vi "NewVSSNavigation.vi"(0 "GoTo Navigation":bool, 1 "a1":dbl=10.0, 2 "VelNearBall":dbl=1.0 format="%#_13g", 3 "output xy":dbl, 4 "IA State Output in":T2, 6 "a3":dbl=15.0, 7 "Penalty Shoot Out?":bool, 8 "PID gains Vel":T1={"proportional gain (Kc)"=0.6, "integral time (Ti, min)"=0.0, "derivative time (Td, min)"=0.0}, 9 "Test Mode":bool, 10 "Debug":bool, 11 "output inc":dbl, 13 "output angle":dbl) -> (14 "IA State Output out":T2)   [LabVIEW 2022 SP3]
uses:
  Vision_class/Old vision/SSL Detection Frame Simple Estimator Cameras VelCmd Folder/Core/AI Input.ctl
  Vision_class/Old vision/Controls/AI Robot.ctl
  Vision_class/Old vision/Controls/Functions Enum.ctl
  Vision_class/Old vision/Controls/AttackerStates.ctl
  Vision_class/Old vision/Controls/PathDests.ctl
  Vision_class/Old vision/Controls/PathDest.ctl
  VSSAttackerStates.ctl
  Vision_class/Old vision/SSL Detection Frame Simple Estimator Cameras VelCmd Folder/Core/AI Ball.ctl
  Vision_class/Old vision/SSL Detection Frame Simple Estimator Cameras VelCmd Folder/Core/Field Size.ctl
  Vision_class/Old vision/SSL Detection Frame Simple Estimator Cameras VelCmd Folder/Core/AI Judge.ctl
  Communication_class/Paths/MessageAI_State Folder/Intel/Command Enum.ctl
  Vision_class/Old vision/SSL Detection Frame Simple Estimator Cameras VelCmd Folder/Util/Events/Events.ctl
  Utilities_class/Utilities.lvclass
  Parameters_class/Project.ctl
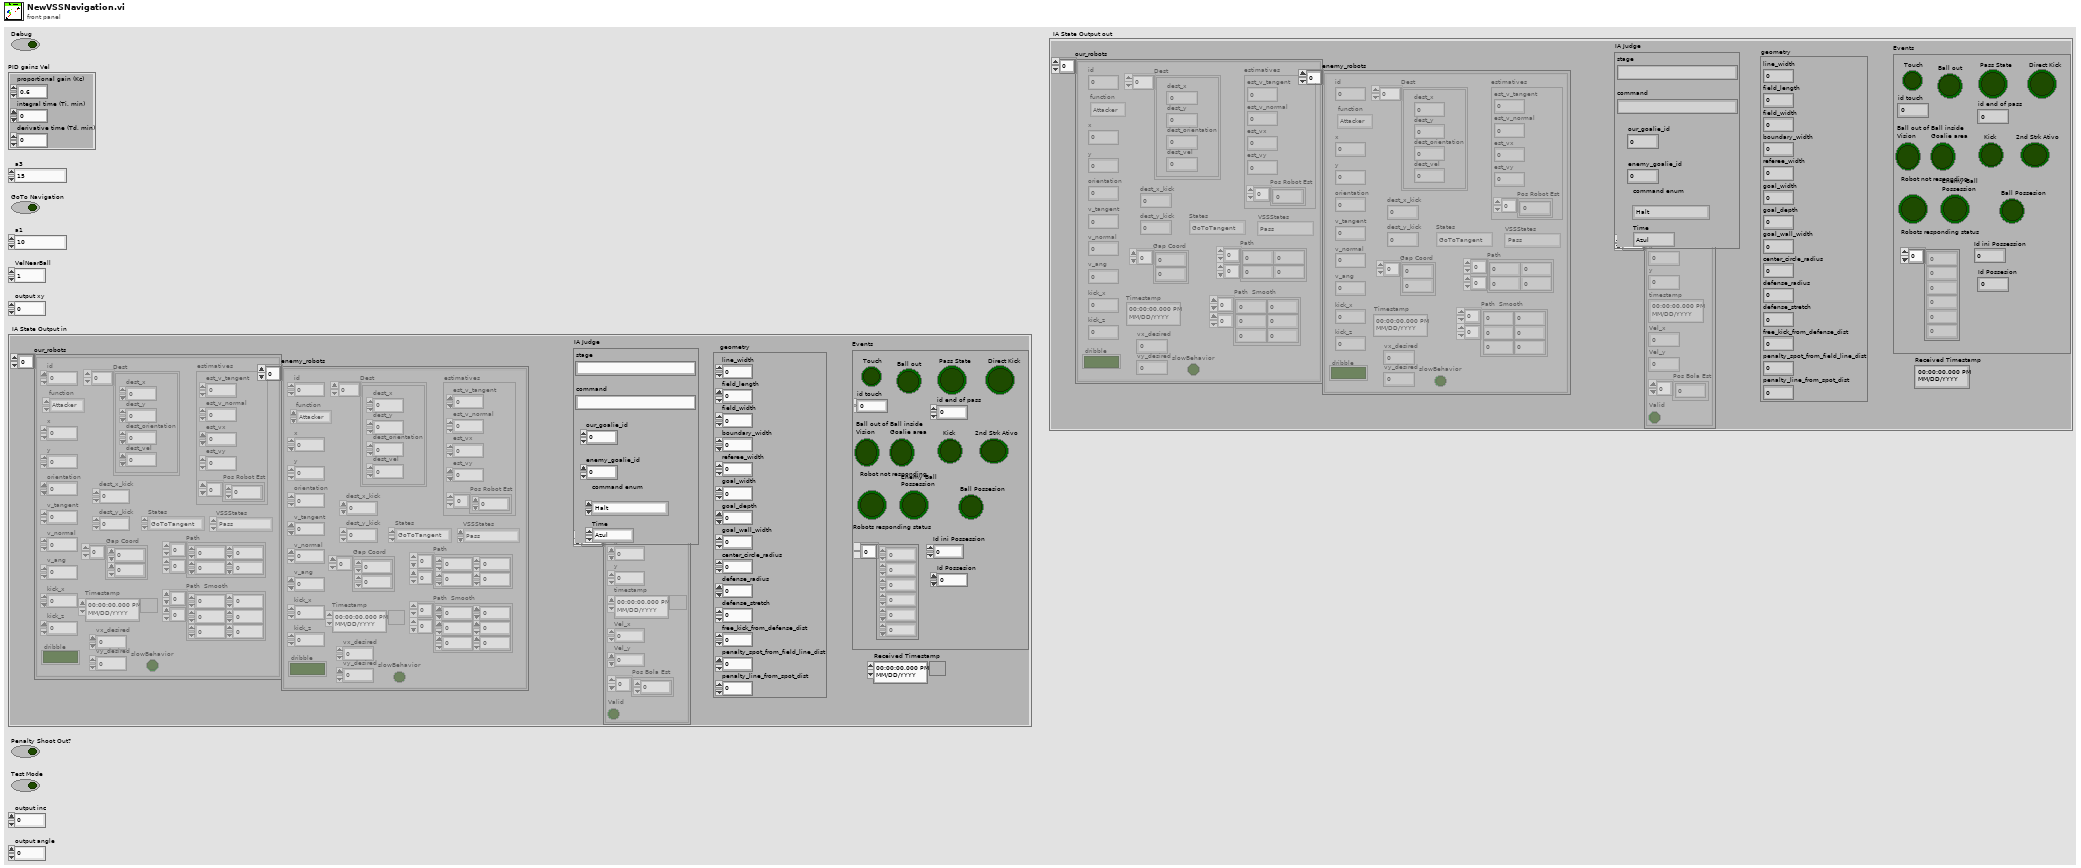
[diagram p1: front panel]
types:
  T1 = cluster{"proportional gain (Kc)":dbl, "integral time (Ti, min)":dbl, "derivative time (Td, min)":dbl}
  T2 = typedef "AI Input.ctl" = cluster{"our_robots":T3[], "enemy_robots":T3[], "balls":T9[], "geometry":T10, "IA Judge":T11, "Received Timestamp":timestamp, "Events":T13}
  T3 = typedef "AI Robot.ctl" = cluster{"id":u32, "function":T4, "x":dbl, "y":dbl, "orientation":dbl, "v_tangent":dbl, "v_normal":dbl, "v_ang":dbl, "kick_x":dbl, "kick_z":dbl, "dribble":bool, "Timestamp":timestamp, "estimatives":cluster{"est_v_tangent":dbl, "est_v_normal":dbl, "est_vx":dbl, "est_vy":dbl, "Pos Robot Est":dbl[]}, "dest_x_kick":dbl, "dest_y_kick":dbl, "Gap Coord":dbl[], "States":T5, "Path ":dbl[][], "Path  Smooth":dbl[][], "Dest":T6, "vx_desired":dbl, "vy_desired":dbl, "slowBehavior":bool, "VSSStates":T8}
  T4 = typedef "Functions Enum.ctl" = enum16{"2nd Striker", "Attacker", "Goalie", "Defender", "Striker", "Goto 0", "Dummy", "Kicker", "ZigZag 0", "ZigZag 1", "ZigZag 2", "ZigZag 3", "ZigZag 4", "ZigZag 5", "ZigZag 6", "ZigZag 7", "ZigZag 8", ""}
  T5 = typedef "AttackerStates.ctl" = enum16{"Pass", "GoToTangent", "BallGetting", "GoToKick", ""}
  T6 = typedef "PathDests.ctl" = T7[]
  T7 = typedef "PathDest.ctl" = cluster{"dest_x":dbl, "dest_y":dbl, "dest_orientation":dbl, "dest_vel":dbl}
  T8 = typedef "VSSAttackerStates.ctl" = enum16{"Pass", "GoToTangent", "BallGetting", "GoToKick", "Rotate anti-clockwise", "Rotate Clockwise", ""}
  T9 = typedef "AI Ball.ctl" = cluster{"x":dbl, "y":dbl, "timestamp":timestamp, "Vel_x":dbl, "Vel_y":dbl, "Pos Bola Est":dbl[], "Valid":bool}
  T10 = typedef "Field Size.ctl" = cluster{"line_width":u32, "field_length":u32, "field_width":u32, "boundary_width":u32, "referee_width":u32, "goal_width":u32, "goal_depth":u32, "goal_wall_width":u32, "center_circle_radius":u32, "defense_radius":u32, "defense_stretch":u32, "free_kick_from_defense_dist":u32, "penalty_spot_from_field_line_dist":u32, "penalty_line_from_spot_dist":u32}
  T11 = typedef "AI Judge.ctl" = cluster{"stage":string, "command":string, "our_goalie_id":dbl, "enemy_goalie_id":dbl, "command enum":T12, "Time":enum16{"Azul", "Amarelo"}}
  T12 = typedef "Command Enum.ctl" = enum16{"Halt", "Stop", "Force Start", "PKA Normal Start", "Prepare Kickoff Ally", "PKE Normal Start", "Prepare Kickoff Enemy", "Prepare Penalty Ally", "PPA Normal Start", "Prepare Penalty Enemy", "PPE Normal Start", "Direct Free Enemy", "Direct Free Ally", "Indirect Free Enemy", "Indirect Free Ally", "Timeout Enemy", "Timeout Ally", "Goal Enemy", "Goal Ally", "Ball Placement Enemy", "Ball Placement Ally", "Normal Half Time", "Extra Time Break", "Extra Half Time", "None", "Post Game"}
  T13 = typedef "Events.ctl" = cluster{"Touch":bool, "Ball out":bool, "id touch":dbl, "Ball out of \nVision":bool, "Ball inside \nGoalie area":bool, "Robot not responding":bool, "Robots responding status":dbl[], "Enemy Ball \nPossession":bool, "Pass State":bool, "id end of pass":dbl, "Kick":bool, "Id ini Possession":dbl, "Ball Possesion":bool, "Id Possesion":dbl, "Direct Kick":bool, "2nd Strk Ativo":bool}
  T14 = typedef "Project.ctl" = enum16{"SSL", "VSS"}
  T15 = cluster{"est_v_tangent":dbl, "est_v_normal":dbl, "est_vx":dbl, "est_vy":dbl, "Pos Robot Est":dbl[]}
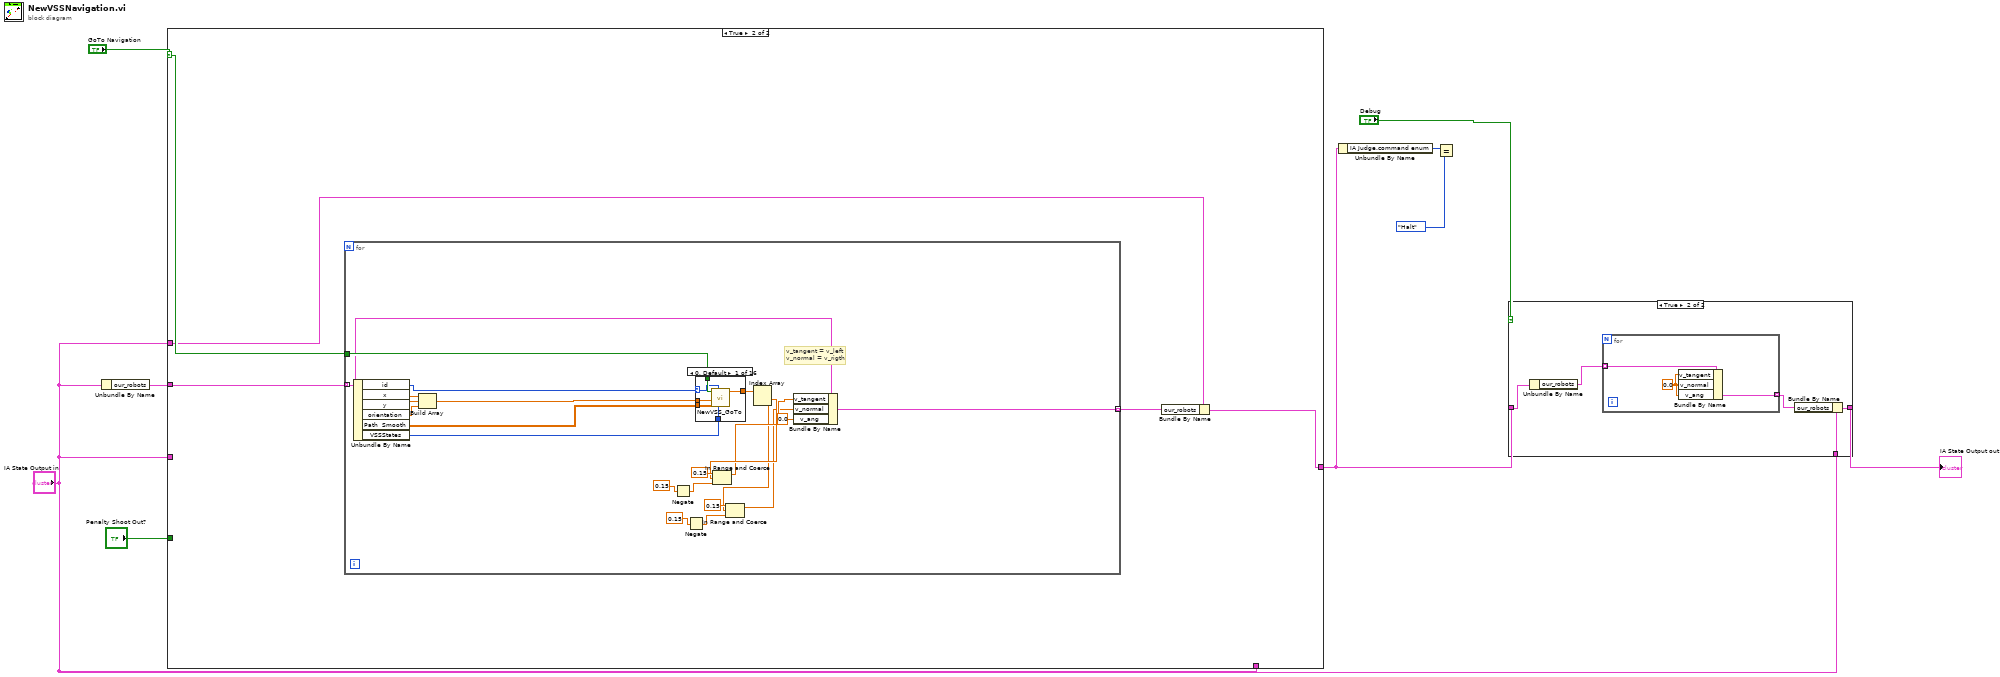
[diagram p0: block diagram]
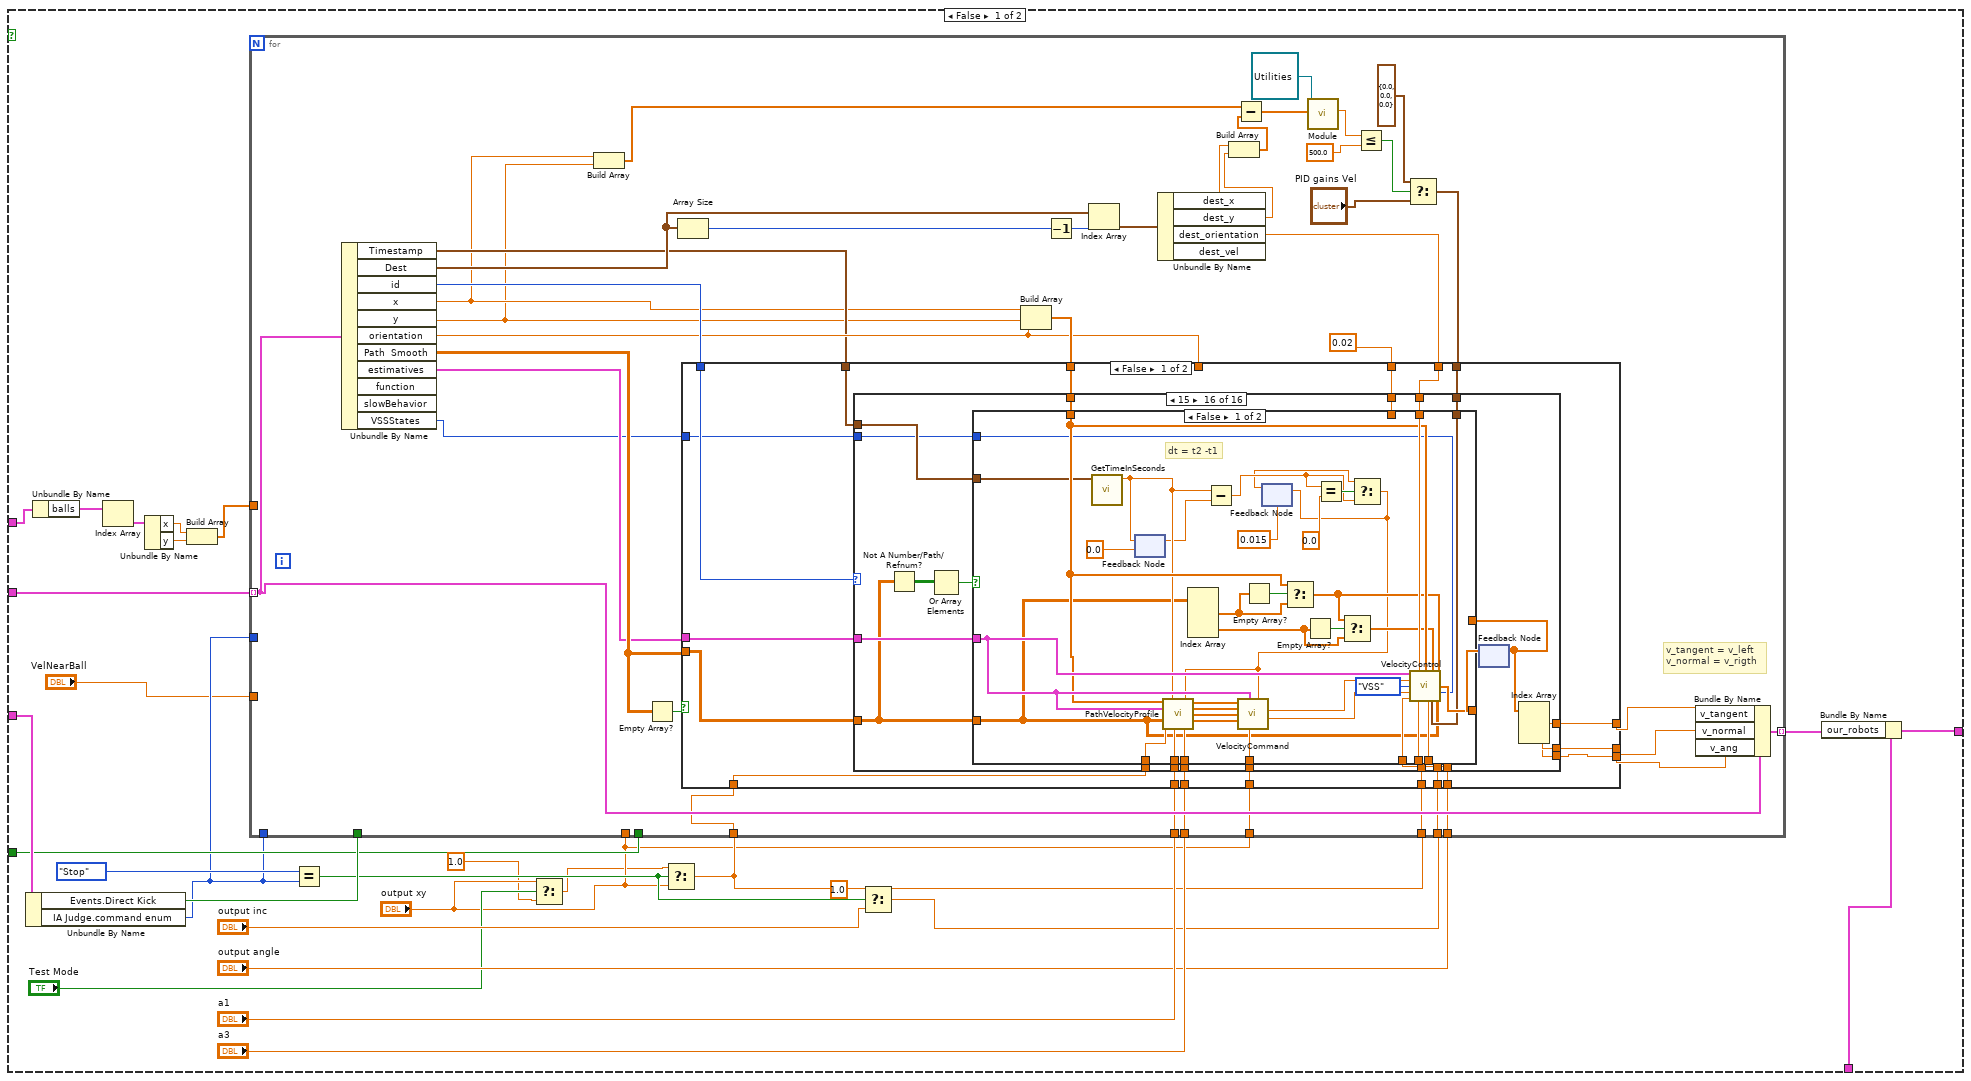
[diagram p2: hidden frame]
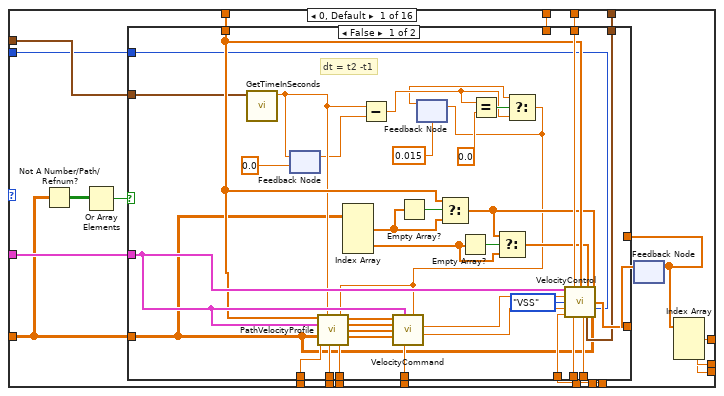
[diagram p3: hidden frame]
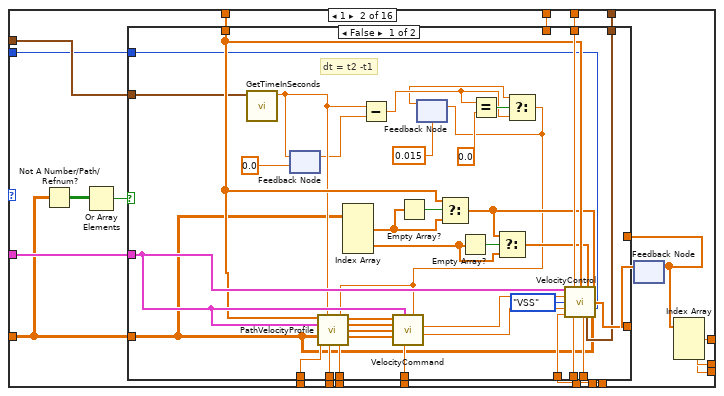
[diagram p5: hidden frame]
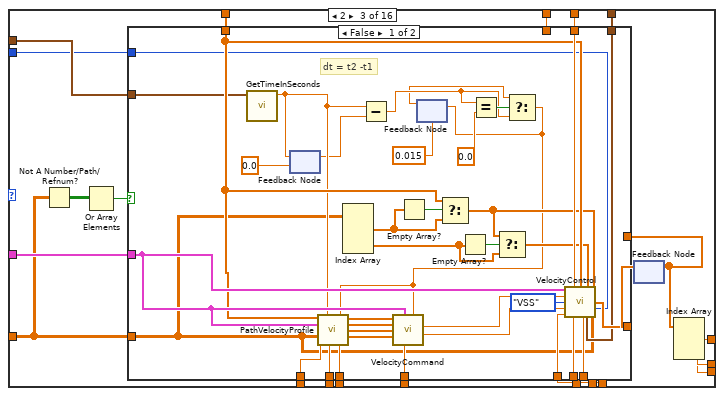
[diagram p7: hidden frame]
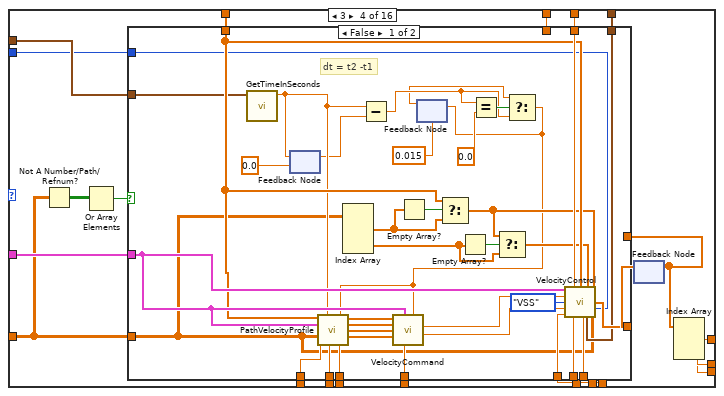
[diagram p9: hidden frame]
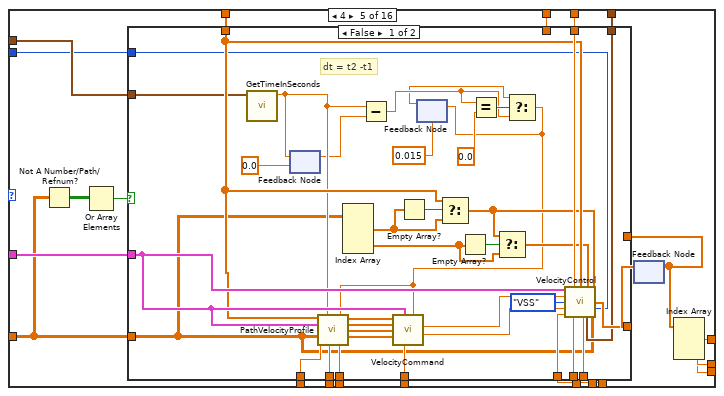
[diagram p11: hidden frame]
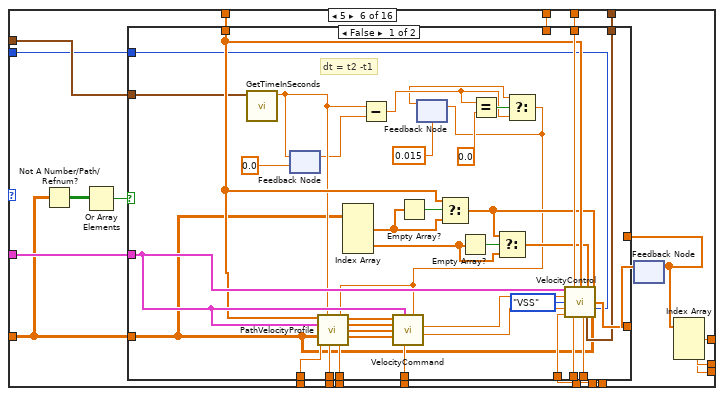
[diagram p13: hidden frame]
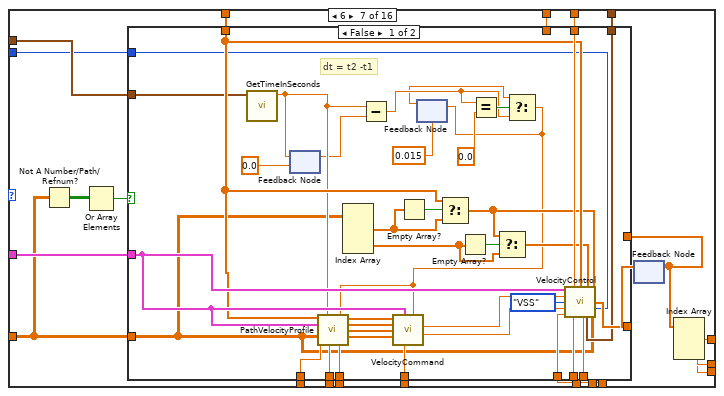
[diagram p15: hidden frame]
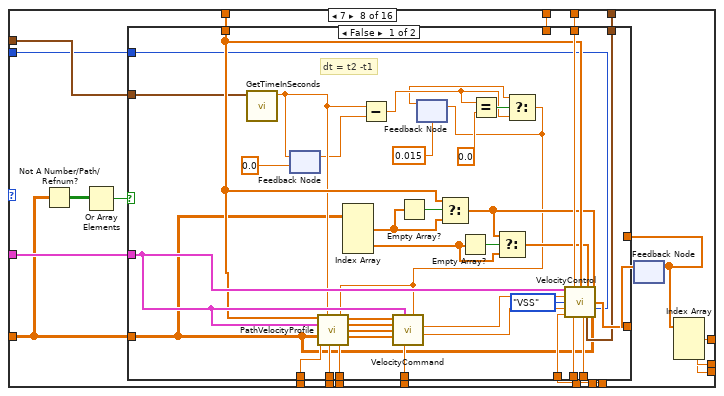
[diagram p17: hidden frame]
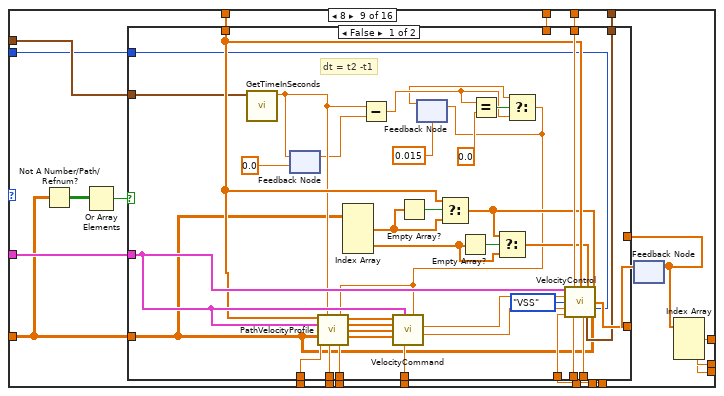
[diagram p19: hidden frame]
diagram:
  n1 = Unbundle By Name("IA State Output in") -> ("our_robots"=w2:T3[])
  n2 = case shown="True" "GoTo Navigation" {
    selector: "GoTo Navigation" -> [_ w1061]
    tunnel: w2 -> [w37 w1062]
    tunnel: [w34 w1060] -> w5
    tunnel: "IA State Output in" -> [w30 _]
    tunnel: "IA State Output in" -> [w35 _]
    tunnel: "IA State Output in" -> [w19 w1059]
    tunnel: "Penalty Shoot Out?" -> [w16 _]
    frame False {
      n3 = Unbundle By Name(w30) -> ("Events.Direct Kick"=w24:bool, "IA Judge.command enum"=w11:T12)
      n4 = Unbundle By Name(w19) -> ("balls"=w23:T9[])
      n5 = Index Array(array=w23) -> (element=w22:T9)  [unwired: 1 in]
      n6 = Unbundle By Name(w22) -> ("x"=w21:dbl, "y"=w20:dbl)
      n7 = Build Array(w21, w20) -> (w18:dbl[])
      n8 = Equal?(x=Command_Enum."Stop", y=w11) -> (x = y?=w17:bool)
      n9 = Select(t="output xy", s="Test Mode", f=1.0 ("t")) -> (s? t:f=w12:dbl)
      n10 = Select(t=w12, s=w17, f="output xy") -> (s? t:f=w28:dbl)
      n11 = Select(t=1.0, s=w17, f="output inc") -> (s? t:f=w26:dbl)
      n12 = for {
        tunnel: w37 -> [w77] mode=indexing
        tunnel: [w76] -> w36 mode=indexing
        tunnel: w28 -> [w38]
        tunnel: "a1" -> [w65]
        tunnel: "a3" -> [w64]
        tunnel: w26 -> [w60]
        tunnel: "output angle" -> [w59]
        tunnel: w28 -> [w58]
        tunnel: w11 -> [_]
        tunnel: w24 -> [_]
        tunnel: w11 -> [_]
        tunnel: w18 -> [_]
        tunnel: w16 -> [_]
        tunnel: "output xy" -> [_]
        tunnel: "output xy" -> [w41]
        tunnel: "VelNearBall" -> [_]
        # "v_tangent = v_left\nv_normal = v_rigth"
        n13 = Unbundle By Name(w77) -> ("Timestamp"=w56:timestamp, "Dest"=w75:T6, "id"=w68:u32, "x"=w54:dbl, "y"=w53:dbl, "orientation"=w63:dbl, "Path  Smooth"=w69:dbl[][], "estimatives"=w66:T15, "VSSStates"=w39:T8)  [unwired: 2 out]
        n14 = Build Array(w54, w53) -> (w49:dbl[])
        n15 = Empty Array?(array=w69) -> (empty?=w70:bool)
        n16 = Array Size(array=w75) -> (size(s)=w74:i32)
        n17 = Build Array(w54, w53, w63) -> (w67:dbl[])
        n18 = Decrement(x=w74) -> (x-1=w73:i32)
        n19 = Index Array(array=w75, index=w73) -> (element=w72:T7)
        n20 = Unbundle By Name(w72) -> ("dest_x"=w52:dbl, "dest_y"=w51:dbl, "dest_orientation"=w71:dbl)  [unwired: 1 out]
        n21 = Build Array(w52, w51) -> (w50:dbl[])
        n22 = Subtract(x=w49, y=w50) -> (x-y=w48:dbl[])
        n23 = call-dynamic "Module.vi"("2D vector"=w48, "Utilities in"=refnum<class "Utilities.lvclass"> refnum) -> ("Modulo"=w46:dbl)  [unwired: 7 in, 2 out]
        n24 = Less Or Equal?(x=w46, y=500.0) -> (x <= y?=w44:bool)
        n25 = Select(t=T1 {"proportional gain (Kc)"=0.0, "integral time (Ti, min)"=0.0, "derivative time (Td, min)"=0.0}, s=w44, f="PID gains Vel") -> (s? t:f=w43:T1)
        n26 = case shown="False" w70 {
          tunnel: [w86 w1057] -> w62
          tunnel: [w85 w1057] -> w61
          tunnel: [w84 w1057] -> w57
          tunnel: w68 -> [w82 _]
          tunnel: w69 -> [w88 _]
          tunnel: w71 -> [w89 _]
          tunnel: w67 -> [w87 _]
          tunnel: w66 -> [w90 _]
          tunnel: w38 -> [w96 _]
          tunnel: w65 -> [w95 _]
          tunnel: w64 -> [w94 _]
          tunnel: w63 -> [_ _]
          tunnel: w60 -> [w93 _]
          tunnel: w59 -> [w92 _]
          tunnel: w58 -> [w91 _]
          tunnel: w56 -> [w83 _]
          tunnel: 0.02 -> [w81 _]
          tunnel: w43 -> [w80 _]
          tunnel: w41 -> [w79 _]
          tunnel: w39 -> [w78 _]
          frame False {
            n27 = case shown="15" w82 {
              tunnel: w96 -> [w118 w178 w238 w298 w358 w418 w478 w538 w598 w658 w718 w778 w838 w898 w958 w1018]
              tunnel: w95 -> [w117 w177 w237 w297 w357 w417 w477 w537 w597 w657 w717 w777 w837 w897 w957 w1017]
              tunnel: w94 -> [w116 w176 w236 w296 w356 w416 w476 w536 w596 w656 w716 w776 w836 w896 w956 w1016]
              tunnel: w93 -> [w115 w175 w235 w295 w355 w415 w475 w535 w595 w655 w715 w775 w835 w895 w955 w1015]
              tunnel: w92 -> [w114 w174 w234 w294 w354 w414 w474 w534 w594 w654 w714 w774 w834 w894 w954 w1014]
              tunnel: w91 -> [w113 w173 w233 w293 w353 w413 w473 w533 w593 w653 w713 w773 w833 w893 w953 w1013]
              tunnel: w90 -> [w112 w172 w232 w292 w352 w412 w472 w532 w592 w652 w712 w772 w832 w892 w952 w1012]
              tunnel: w89 -> [w111 w171 w231 w291 w351 w411 w471 w531 w591 w651 w711 w771 w831 w891 w951 w1011]
              tunnel: w88 -> [w103 w163 w223 w283 w343 w403 w463 w523 w583 w643 w703 w763 w823 w883 w943 w1003]
              tunnel: w87 -> [w110 w170 w230 w290 w350 w410 w470 w530 w590 w650 w710 w770 w830 w890 w950 w1010]
              tunnel: [w109 w169 w229 w289 w349 w409 w469 w529 w589 w649 w709 w769 w829 w889 w949 w1009] -> w86
              tunnel: [w108 w168 w228 w288 w348 w408 w468 w528 w588 w648 w708 w768 w828 w888 w948 w1008] -> w85
              tunnel: [w107 w167 w227 w287 w347 w407 w467 w527 w587 w647 w707 w767 w827 w887 w947 w1007] -> w84
              tunnel: w83 -> [w106 w166 w226 w286 w346 w406 w466 w526 w586 w646 w706 w766 w826 w886 w946 w1006]
              tunnel: w81 -> [w100 w160 w220 w280 w340 w400 w460 w520 w580 w640 w700 w760 w820 w880 w940 w1000]
              tunnel: w80 -> [w99 w159 w219 w279 w339 w399 w459 w519 w579 w639 w699 w759 w819 w879 w939 w999]
              tunnel: w79 -> [w98 w158 w218 w278 w338 w398 w458 w518 w578 w638 w698 w758 w818 w878 w938 w998]
              tunnel: w78 -> [w97 w157 w217 w277 w337 w397 w457 w517 w577 w637 w697 w757 w817 w877 w937 w997]
              frame 0, Default {
                n28 = Not A Number/Path/Refnum?(number/path/refnum=w103) -> (NaN/Path/Refnum?=w102:bool[][])
                n29 = Or Array Elements(Boolean array=w102) -> (logical OR=w101:bool)
                n30 = feedback #1() -> (w104:dbl[])  [unwired: 1 in]
                n31 = case shown="False" w101 {
                  tunnel: w118 -> [w155 _]
                  tunnel: w117 -> [w154 _]
                  tunnel: w116 -> [w153 _]
                  tunnel: w115 -> [w152 _]
                  tunnel: w114 -> [w151 _]
                  tunnel: w113 -> [w150 _]
                  tunnel: w112 -> [w149 _]
                  tunnel: w111 -> [w148 _]
                  tunnel: w103 -> [w120 _]
                  tunnel: w110 -> [w147 _]
                  tunnel: [w146 w156] -> w105
                  tunnel: w106 -> [w133 _]
                  tunnel: w104 -> [_ w156]
                  tunnel: w100 -> [_ _]
                  tunnel: w99 -> [w124 _]
                  tunnel: w98 -> [w122 _]
                  tunnel: w97 -> [w119 _]
                  frame False {
                    # "dt = t2 -t1"
                    n32 = call "GetTimeInSeconds.vi"("Timestamp"=w133) -> ("Numeric"=w127:dbl)  [unwired: 10 in]
                    n33 = feedback-in #2(w127) -> ()
                    n34 = feedback #2(0.0 ("Numeric")) -> (w126:dbl)
                    n35 = Index Array(array=w120) -> (element #1=w135:dbl[], element #2=w138:dbl[])  [unwired: 4 in]
                    n36 = Subtract(x=w127, y=w126) -> (x-y=w129:dbl)
                    n37 = Empty Array?(array=w135) -> (empty?=w136:bool)
                    n38 = feedback #3(0.015 ("Numeric")) -> (w128:dbl)
                    n39 = Select(t=w147, s=w136, f=w135) -> (s? t:f=w134:dbl[])
                    n40 = Empty Array?(array=w138) -> (empty?=w139:bool)
                    n41 = Equal?(x=w129, y=0.0) -> (x = y?=w132:bool)
                    n42 = Select(t=w134, s=w139, f=w138) -> (s? t:f=w137:dbl[])
                    n43 = Select(t=w128, s=w132, f=w129) -> (s? t:f=w123:dbl)
                    n44 = call "PathVelocityProfile.vi"("Pose"=w147, "time"=w127, "intervalo"=w123, "estimatives"=w149, "Path  Smooth"=w120, "V_max"=w155, "Accel"=w154, "DesAccel"=w153) -> ("Time X"=w145:dbl[], "Velocities X"=w144:dbl[], "Time Y"=w143:dbl[], "Velocities Y"=w142:dbl[])  [unwired: 4 in]
                    n45 = call "VelocityCommand.vi"("intervalo"=w123, "MaxOutputXY"=w122, "estimatives"=w149, "Velocities Y"=w142, "Time Y"=w143, "Velocities X"=w144, "Time X"=w145) -> ("Vy"=w141:dbl, "Vx"=w140:dbl)  [unwired: 3 in]
                    n46 = feedback-in #3(w123) -> ()
                    n47 = call "VelocityControl.vi"("estimatives"=w149, "Dest_orientation"=w148, "Position"=w147, "Waypoint 1"=w137, "Waypoint 0"=w134, "Vx"=w140, "Project"=Project."VSS", "Vy"=w141, "VSSStates"=w119, "output xy"=w150, "output inc"=w152, "output angle"=w151, "PID gains Vel"=w124, "Path  Smooth"=w120) -> ("Output Velocity"=w146:dbl[])  [unwired: 1 in]
                  }
                  frame True {
                  }
                }
                n48 = feedback-in #1(w105) -> ()
                n49 = Index Array(array=w104) -> (element #1=w109:dbl, element #2=w108:dbl, element #3=w107:dbl)  [unwired: 3 in]
              }
              frame 1 {
                n50 = Not A Number/Path/Refnum?(number/path/refnum=w163) -> (NaN/Path/Refnum?=w162:bool[][])
                n51 = Or Array Elements(Boolean array=w162) -> (logical OR=w161:bool)
                n52 = feedback #4() -> (w164:dbl[])  [unwired: 1 in]
                n53 = case shown="False" w161 {
                  tunnel: w178 -> [w215 _]
                  tunnel: w177 -> [w214 _]
                  tunnel: w176 -> [w213 _]
                  tunnel: w175 -> [w212 _]
                  tunnel: w174 -> [w211 _]
                  tunnel: w173 -> [w210 _]
                  tunnel: w172 -> [w209 _]
                  tunnel: w171 -> [w208 _]
                  tunnel: w163 -> [w180 _]
                  tunnel: w170 -> [w207 _]
                  tunnel: [w206 w216] -> w165
                  tunnel: w166 -> [w193 _]
                  tunnel: w164 -> [_ w216]
                  tunnel: w160 -> [_ _]
                  tunnel: w159 -> [w184 _]
                  tunnel: w158 -> [w182 _]
                  tunnel: w157 -> [w179 _]
                  frame False {
                    # "dt = t2 -t1"
                    n54 = call "GetTimeInSeconds.vi"("Timestamp"=w193) -> ("Numeric"=w187:dbl)  [unwired: 10 in]
                    n55 = feedback-in #5(w187) -> ()
                    n56 = feedback #5(0.0 ("Numeric")) -> (w186:dbl)
                    n57 = Index Array(array=w180) -> (element #1=w195:dbl[], element #2=w198:dbl[])  [unwired: 4 in]
                    n58 = Subtract(x=w187, y=w186) -> (x-y=w189:dbl)
                    n59 = Empty Array?(array=w195) -> (empty?=w196:bool)
                    n60 = feedback #6(0.015 ("Numeric")) -> (w188:dbl)
                    n61 = Select(t=w207, s=w196, f=w195) -> (s? t:f=w194:dbl[])
                    n62 = Empty Array?(array=w198) -> (empty?=w199:bool)
                    n63 = Equal?(x=w189, y=0.0) -> (x = y?=w192:bool)
                    n64 = Select(t=w194, s=w199, f=w198) -> (s? t:f=w197:dbl[])
                    n65 = Select(t=w188, s=w192, f=w189) -> (s? t:f=w183:dbl)
                    n66 = call "PathVelocityProfile.vi"("Pose"=w207, "time"=w187, "intervalo"=w183, "estimatives"=w209, "Path  Smooth"=w180, "V_max"=w215, "Accel"=w214, "DesAccel"=w213) -> ("Time X"=w205:dbl[], "Velocities X"=w204:dbl[], "Time Y"=w203:dbl[], "Velocities Y"=w202:dbl[])  [unwired: 4 in]
                    n67 = call "VelocityCommand.vi"("intervalo"=w183, "MaxOutputXY"=w182, "estimatives"=w209, "Velocities Y"=w202, "Time Y"=w203, "Velocities X"=w204, "Time X"=w205) -> ("Vy"=w201:dbl, "Vx"=w200:dbl)  [unwired: 3 in]
                    n68 = feedback-in #6(w183) -> ()
                    n69 = call "VelocityControl.vi"("estimatives"=w209, "Dest_orientation"=w208, "Position"=w207, "Waypoint 1"=w197, "Waypoint 0"=w194, "Vx"=w200, "Project"=Project."VSS", "Vy"=w201, "VSSStates"=w179, "output xy"=w210, "output inc"=w212, "output angle"=w211, "PID gains Vel"=w184, "Path  Smooth"=w180) -> ("Output Velocity"=w206:dbl[])  [unwired: 1 in]
                  }
                  frame True {
                  }
                }
                n70 = feedback-in #4(w165) -> ()
                n71 = Index Array(array=w164) -> (element #1=w169:dbl, element #2=w168:dbl, element #3=w167:dbl)  [unwired: 3 in]
              }
              frame 2 {
                n72 = Not A Number/Path/Refnum?(number/path/refnum=w223) -> (NaN/Path/Refnum?=w222:bool[][])
                n73 = Or Array Elements(Boolean array=w222) -> (logical OR=w221:bool)
                n74 = feedback #7() -> (w224:dbl[])  [unwired: 1 in]
                n75 = case shown="False" w221 {
                  tunnel: w238 -> [w275 _]
                  tunnel: w237 -> [w274 _]
                  tunnel: w236 -> [w273 _]
                  tunnel: w235 -> [w272 _]
                  tunnel: w234 -> [w271 _]
                  tunnel: w233 -> [w270 _]
                  tunnel: w232 -> [w269 _]
                  tunnel: w231 -> [w268 _]
                  tunnel: w223 -> [w240 _]
                  tunnel: w230 -> [w267 _]
                  tunnel: [w266 w276] -> w225
                  tunnel: w226 -> [w253 _]
                  tunnel: w224 -> [_ w276]
                  tunnel: w220 -> [_ _]
                  tunnel: w219 -> [w244 _]
                  tunnel: w218 -> [w242 _]
                  tunnel: w217 -> [w239 _]
                  frame False {
                    # "dt = t2 -t1"
                    n76 = call "GetTimeInSeconds.vi"("Timestamp"=w253) -> ("Numeric"=w247:dbl)  [unwired: 10 in]
                    n77 = feedback-in #8(w247) -> ()
                    n78 = feedback #8(0.0 ("Numeric")) -> (w246:dbl)
                    n79 = Index Array(array=w240) -> (element #1=w255:dbl[], element #2=w258:dbl[])  [unwired: 4 in]
                    n80 = Subtract(x=w247, y=w246) -> (x-y=w249:dbl)
                    n81 = Empty Array?(array=w255) -> (empty?=w256:bool)
                    n82 = feedback #9(0.015 ("Numeric")) -> (w248:dbl)
                    n83 = Select(t=w267, s=w256, f=w255) -> (s? t:f=w254:dbl[])
                    n84 = Empty Array?(array=w258) -> (empty?=w259:bool)
                    n85 = Equal?(x=w249, y=0.0) -> (x = y?=w252:bool)
                    n86 = Select(t=w254, s=w259, f=w258) -> (s? t:f=w257:dbl[])
                    n87 = Select(t=w248, s=w252, f=w249) -> (s? t:f=w243:dbl)
                    n88 = call "PathVelocityProfile.vi"("Pose"=w267, "time"=w247, "intervalo"=w243, "estimatives"=w269, "Path  Smooth"=w240, "V_max"=w275, "Accel"=w274, "DesAccel"=w273) -> ("Time X"=w265:dbl[], "Velocities X"=w264:dbl[], "Time Y"=w263:dbl[], "Velocities Y"=w262:dbl[])  [unwired: 4 in]
                    n89 = call "VelocityCommand.vi"("intervalo"=w243, "MaxOutputXY"=w242, "estimatives"=w269, "Velocities Y"=w262, "Time Y"=w263, "Velocities X"=w264, "Time X"=w265) -> ("Vy"=w261:dbl, "Vx"=w260:dbl)  [unwired: 3 in]
                    n90 = feedback-in #9(w243) -> ()
                    n91 = call "VelocityControl.vi"("estimatives"=w269, "Dest_orientation"=w268, "Position"=w267, "Waypoint 1"=w257, "Waypoint 0"=w254, "Vx"=w260, "Project"=Project."VSS", "Vy"=w261, "VSSStates"=w239, "output xy"=w270, "output inc"=w272, "output angle"=w271, "PID gains Vel"=w244, "Path  Smooth"=w240) -> ("Output Velocity"=w266:dbl[])  [unwired: 1 in]
                  }
                  frame True {
                  }
                }
                n92 = feedback-in #7(w225) -> ()
                n93 = Index Array(array=w224) -> (element #1=w229:dbl, element #2=w228:dbl, element #3=w227:dbl)  [unwired: 3 in]
              }
              frame 3 {
                n94 = Not A Number/Path/Refnum?(number/path/refnum=w283) -> (NaN/Path/Refnum?=w282:bool[][])
                n95 = Or Array Elements(Boolean array=w282) -> (logical OR=w281:bool)
                n96 = feedback #10() -> (w284:dbl[])  [unwired: 1 in]
                n97 = case shown="False" w281 {
                  tunnel: w298 -> [w335 _]
                  tunnel: w297 -> [w334 _]
                  tunnel: w296 -> [w333 _]
                  tunnel: w295 -> [w332 _]
                  tunnel: w294 -> [w331 _]
                  tunnel: w293 -> [w330 _]
                  tunnel: w292 -> [w329 _]
                  tunnel: w291 -> [w328 _]
                  tunnel: w283 -> [w300 _]
                  tunnel: w290 -> [w327 _]
                  tunnel: [w326 w336] -> w285
                  tunnel: w286 -> [w313 _]
                  tunnel: w284 -> [_ w336]
                  tunnel: w280 -> [_ _]
                  tunnel: w279 -> [w304 _]
                  tunnel: w278 -> [w302 _]
                  tunnel: w277 -> [w299 _]
                  frame False {
                    # "dt = t2 -t1"
                    n98 = call "GetTimeInSeconds.vi"("Timestamp"=w313) -> ("Numeric"=w307:dbl)  [unwired: 10 in]
                    n99 = feedback-in #11(w307) -> ()
                    n100 = feedback #11(0.0 ("Numeric")) -> (w306:dbl)
                    n101 = Index Array(array=w300) -> (element #1=w315:dbl[], element #2=w318:dbl[])  [unwired: 4 in]
                    n102 = Subtract(x=w307, y=w306) -> (x-y=w309:dbl)
                    n103 = Empty Array?(array=w315) -> (empty?=w316:bool)
                    n104 = feedback #12(0.015 ("Numeric")) -> (w308:dbl)
                    n105 = Select(t=w327, s=w316, f=w315) -> (s? t:f=w314:dbl[])
                    n106 = Empty Array?(array=w318) -> (empty?=w319:bool)
                    n107 = Equal?(x=w309, y=0.0) -> (x = y?=w312:bool)
                    n108 = Select(t=w314, s=w319, f=w318) -> (s? t:f=w317:dbl[])
                    n109 = Select(t=w308, s=w312, f=w309) -> (s? t:f=w303:dbl)
                    n110 = call "PathVelocityProfile.vi"("Pose"=w327, "time"=w307, "intervalo"=w303, "estimatives"=w329, "Path  Smooth"=w300, "V_max"=w335, "Accel"=w334, "DesAccel"=w333) -> ("Time X"=w325:dbl[], "Velocities X"=w324:dbl[], "Time Y"=w323:dbl[], "Velocities Y"=w322:dbl[])  [unwired: 4 in]
                    n111 = call "VelocityCommand.vi"("intervalo"=w303, "MaxOutputXY"=w302, "estimatives"=w329, "Velocities Y"=w322, "Time Y"=w323, "Velocities X"=w324, "Time X"=w325) -> ("Vy"=w321:dbl, "Vx"=w320:dbl)  [unwired: 3 in]
                    n112 = feedback-in #12(w303) -> ()
                    n113 = call "VelocityControl.vi"("estimatives"=w329, "Dest_orientation"=w328, "Position"=w327, "Waypoint 1"=w317, "Waypoint 0"=w314, "Vx"=w320, "Project"=Project."VSS", "Vy"=w321, "VSSStates"=w299, "output xy"=w330, "output inc"=w332, "output angle"=w331, "PID gains Vel"=w304, "Path  Smooth"=w300) -> ("Output Velocity"=w326:dbl[])  [unwired: 1 in]
                  }
                  frame True {
                  }
                }
                n114 = feedback-in #10(w285) -> ()
                n115 = Index Array(array=w284) -> (element #1=w289:dbl, element #2=w288:dbl, element #3=w287:dbl)  [unwired: 3 in]
              }
              frame 4 {
                n116 = Not A Number/Path/Refnum?(number/path/refnum=w343) -> (NaN/Path/Refnum?=w342:bool[][])
                n117 = Or Array Elements(Boolean array=w342) -> (logical OR=w341:bool)
                n118 = feedback #13() -> (w344:dbl[])  [unwired: 1 in]
                n119 = case shown="False" w341 {
                  tunnel: w358 -> [w395 _]
                  tunnel: w357 -> [w394 _]
                  tunnel: w356 -> [w393 _]
                  tunnel: w355 -> [w392 _]
                  tunnel: w354 -> [w391 _]
                  tunnel: w353 -> [w390 _]
                  tunnel: w352 -> [w389 _]
                  tunnel: w351 -> [w388 _]
                  tunnel: w343 -> [w360 _]
                  tunnel: w350 -> [w387 _]
                  tunnel: [w386 w396] -> w345
                  tunnel: w346 -> [w373 _]
                  tunnel: w344 -> [_ w396]
                  tunnel: w340 -> [_ _]
                  tunnel: w339 -> [w364 _]
                  tunnel: w338 -> [w362 _]
                  tunnel: w337 -> [w359 _]
                  frame False {
                    # "dt = t2 -t1"
                    n120 = call "GetTimeInSeconds.vi"("Timestamp"=w373) -> ("Numeric"=w367:dbl)  [unwired: 10 in]
                    n121 = feedback-in #14(w367) -> ()
                    n122 = feedback #14(0.0 ("Numeric")) -> (w366:dbl)
                    n123 = Index Array(array=w360) -> (element #1=w375:dbl[], element #2=w378:dbl[])  [unwired: 4 in]
                    n124 = Subtract(x=w367, y=w366) -> (x-y=w369:dbl)
                    n125 = Empty Array?(array=w375) -> (empty?=w376:bool)
                    n126 = feedback #15(0.015 ("Numeric")) -> (w368:dbl)
                    n127 = Select(t=w387, s=w376, f=w375) -> (s? t:f=w374:dbl[])
                    n128 = Empty Array?(array=w378) -> (empty?=w379:bool)
                    n129 = Equal?(x=w369, y=0.0) -> (x = y?=w372:bool)
                    n130 = Select(t=w374, s=w379, f=w378) -> (s? t:f=w377:dbl[])
                    n131 = Select(t=w368, s=w372, f=w369) -> (s? t:f=w363:dbl)
                    n132 = call "PathVelocityProfile.vi"("Pose"=w387, "time"=w367, "intervalo"=w363, "estimatives"=w389, "Path  Smooth"=w360, "V_max"=w395, "Accel"=w394, "DesAccel"=w393) -> ("Time X"=w385:dbl[], "Velocities X"=w384:dbl[], "Time Y"=w383:dbl[], "Velocities Y"=w382:dbl[])  [unwired: 4 in]
                    n133 = call "VelocityCommand.vi"("intervalo"=w363, "MaxOutputXY"=w362, "estimatives"=w389, "Velocities Y"=w382, "Time Y"=w383, "Velocities X"=w384, "Time X"=w385) -> ("Vy"=w381:dbl, "Vx"=w380:dbl)  [unwired: 3 in]
                    n134 = feedback-in #15(w363) -> ()
                    n135 = call "VelocityControl.vi"("estimatives"=w389, "Dest_orientation"=w388, "Position"=w387, "Waypoint 1"=w377, "Waypoint 0"=w374, "Vx"=w380, "Project"=Project."VSS", "Vy"=w381, "VSSStates"=w359, "output xy"=w390, "output inc"=w392, "output angle"=w391, "PID gains Vel"=w364, "Path  Smooth"=w360) -> ("Output Velocity"=w386:dbl[])  [unwired: 1 in]
                  }
                  frame True {
                  }
                }
                n136 = feedback-in #13(w345) -> ()
                n137 = Index Array(array=w344) -> (element #1=w349:dbl, element #2=w348:dbl, element #3=w347:dbl)  [unwired: 3 in]
              }
              frame 5 {
                n138 = Not A Number/Path/Refnum?(number/path/refnum=w403) -> (NaN/Path/Refnum?=w402:bool[][])
                n139 = Or Array Elements(Boolean array=w402) -> (logical OR=w401:bool)
                n140 = feedback #16() -> (w404:dbl[])  [unwired: 1 in]
                n141 = case shown="False" w401 {
                  tunnel: w418 -> [w455 _]
                  tunnel: w417 -> [w454 _]
                  tunnel: w416 -> [w453 _]
                  tunnel: w415 -> [w452 _]
                  tunnel: w414 -> [w451 _]
                  tunnel: w413 -> [w450 _]
                  tunnel: w412 -> [w449 _]
                  tunnel: w411 -> [w448 _]
                  tunnel: w403 -> [w420 _]
                  tunnel: w410 -> [w447 _]
                  tunnel: [w446 w456] -> w405
                  tunnel: w406 -> [w433 _]
                  tunnel: w404 -> [_ w456]
                  tunnel: w400 -> [_ _]
                  tunnel: w399 -> [w424 _]
                  tunnel: w398 -> [w422 _]
                  tunnel: w397 -> [w419 _]
                  frame False {
                    # "dt = t2 -t1"
                    n142 = call "GetTimeInSeconds.vi"("Timestamp"=w433) -> ("Numeric"=w427:dbl)  [unwired: 10 in]
                    n143 = feedback-in #17(w427) -> ()
                    n144 = feedback #17(0.0 ("Numeric")) -> (w426:dbl)
                    n145 = Index Array(array=w420) -> (element #1=w435:dbl[], element #2=w438:dbl[])  [unwired: 4 in]
                    n146 = Subtract(x=w427, y=w426) -> (x-y=w429:dbl)
                    n147 = Empty Array?(array=w435) -> (empty?=w436:bool)
                    n148 = feedback #18(0.015 ("Numeric")) -> (w428:dbl)
                    n149 = Select(t=w447, s=w436, f=w435) -> (s? t:f=w434:dbl[])
                    n150 = Empty Array?(array=w438) -> (empty?=w439:bool)
                    n151 = Equal?(x=w429, y=0.0) -> (x = y?=w432:bool)
                    n152 = Select(t=w434, s=w439, f=w438) -> (s? t:f=w437:dbl[])
                    n153 = Select(t=w428, s=w432, f=w429) -> (s? t:f=w423:dbl)
                    n154 = call "PathVelocityProfile.vi"("Pose"=w447, "time"=w427, "intervalo"=w423, "estimatives"=w449, "Path  Smooth"=w420, "V_max"=w455, "Accel"=w454, "DesAccel"=w453) -> ("Time X"=w445:dbl[], "Velocities X"=w444:dbl[], "Time Y"=w443:dbl[], "Velocities Y"=w442:dbl[])  [unwired: 4 in]
                    n155 = call "VelocityCommand.vi"("intervalo"=w423, "MaxOutputXY"=w422, "estimatives"=w449, "Velocities Y"=w442, "Time Y"=w443, "Velocities X"=w444, "Time X"=w445) -> ("Vy"=w441:dbl, "Vx"=w440:dbl)  [unwired: 3 in]
                    n156 = feedback-in #18(w423) -> ()
                    n157 = call "VelocityControl.vi"("estimatives"=w449, "Dest_orientation"=w448, "Position"=w447, "Waypoint 1"=w437, "Waypoint 0"=w434, "Vx"=w440, "Project"=Project."VSS", "Vy"=w441, "VSSStates"=w419, "output xy"=w450, "output inc"=w452, "output angle"=w451, "PID gains Vel"=w424, "Path  Smooth"=w420) -> ("Output Velocity"=w446:dbl[])  [unwired: 1 in]
                  }
                  frame True {
                  }
                }
                n158 = feedback-in #16(w405) -> ()
                n159 = Index Array(array=w404) -> (element #1=w409:dbl, element #2=w408:dbl, element #3=w407:dbl)  [unwired: 3 in]
              }
              frame 6 {
                n160 = Not A Number/Path/Refnum?(number/path/refnum=w463) -> (NaN/Path/Refnum?=w462:bool[][])
                n161 = Or Array Elements(Boolean array=w462) -> (logical OR=w461:bool)
                n162 = feedback #19() -> (w464:dbl[])  [unwired: 1 in]
                n163 = case shown="False" w461 {
                  tunnel: w478 -> [w515 _]
                  tunnel: w477 -> [w514 _]
                  tunnel: w476 -> [w513 _]
                  tunnel: w475 -> [w512 _]
                  tunnel: w474 -> [w511 _]
                  tunnel: w473 -> [w510 _]
                  tunnel: w472 -> [w509 _]
                  tunnel: w471 -> [w508 _]
                  tunnel: w463 -> [w480 _]
                  tunnel: w470 -> [w507 _]
                  tunnel: [w506 w516] -> w465
                  tunnel: w466 -> [w493 _]
                  tunnel: w464 -> [_ w516]
                  tunnel: w460 -> [_ _]
                  tunnel: w459 -> [w484 _]
                  tunnel: w458 -> [w482 _]
                  tunnel: w457 -> [w479 _]
                  frame False {
                    # "dt = t2 -t1"
                    n164 = call "GetTimeInSeconds.vi"("Timestamp"=w493) -> ("Numeric"=w487:dbl)  [unwired: 10 in]
                    n165 = feedback-in #20(w487) -> ()
                    n166 = feedback #20(0.0 ("Numeric")) -> (w486:dbl)
                    n167 = Index Array(array=w480) -> (element #1=w495:dbl[], element #2=w498:dbl[])  [unwired: 4 in]
                    n168 = Subtract(x=w487, y=w486) -> (x-y=w489:dbl)
                    n169 = Empty Array?(array=w495) -> (empty?=w496:bool)
                    n170 = feedback #21(0.015 ("Numeric")) -> (w488:dbl)
                    n171 = Select(t=w507, s=w496, f=w495) -> (s? t:f=w494:dbl[])
                    n172 = Empty Array?(array=w498) -> (empty?=w499:bool)
                    n173 = Equal?(x=w489, y=0.0) -> (x = y?=w492:bool)
                    n174 = Select(t=w494, s=w499, f=w498) -> (s? t:f=w497:dbl[])
                    n175 = Select(t=w488, s=w492, f=w489) -> (s? t:f=w483:dbl)
                    n176 = call "PathVelocityProfile.vi"("Pose"=w507, "time"=w487, "intervalo"=w483, "estimatives"=w509, "Path  Smooth"=w480, "V_max"=w515, "Accel"=w514, "DesAccel"=w513) -> ("Time X"=w505:dbl[], "Velocities X"=w504:dbl[], "Time Y"=w503:dbl[], "Velocities Y"=w502:dbl[])  [unwired: 4 in]
                    n177 = call "VelocityCommand.vi"("intervalo"=w483, "MaxOutputXY"=w482, "estimatives"=w509, "Velocities Y"=w502, "Time Y"=w503, "Velocities X"=w504, "Time X"=w505) -> ("Vy"=w501:dbl, "Vx"=w500:dbl)  [unwired: 3 in]
                    n178 = feedback-in #21(w483) -> ()
                    n179 = call "VelocityControl.vi"("estimatives"=w509, "Dest_orientation"=w508, "Position"=w507, "Waypoint 1"=w497, "Waypoint 0"=w494, "Vx"=w500, "Project"=Project."VSS", "Vy"=w501, "VSSStates"=w479, "output xy"=w510, "output inc"=w512, "output angle"=w511, "PID gains Vel"=w484, "Path  Smooth"=w480) -> ("Output Velocity"=w506:dbl[])  [unwired: 1 in]
                  }
                  frame True {
                  }
                }
                n180 = feedback-in #19(w465) -> ()
                n181 = Index Array(array=w464) -> (element #1=w469:dbl, element #2=w468:dbl, element #3=w467:dbl)  [unwired: 3 in]
              }
              frame 7 {
                n182 = Not A Number/Path/Refnum?(number/path/refnum=w523) -> (NaN/Path/Refnum?=w522:bool[][])
                n183 = Or Array Elements(Boolean array=w522) -> (logical OR=w521:bool)
                n184 = feedback #22() -> (w524:dbl[])  [unwired: 1 in]
                n185 = case shown="False" w521 {
                  tunnel: w538 -> [w575 _]
                  tunnel: w537 -> [w574 _]
                  tunnel: w536 -> [w573 _]
                  tunnel: w535 -> [w572 _]
                  tunnel: w534 -> [w571 _]
                  tunnel: w533 -> [w570 _]
                  tunnel: w532 -> [w569 _]
                  tunnel: w531 -> [w568 _]
                  tunnel: w523 -> [w540 _]
                  tunnel: w530 -> [w567 _]
                  tunnel: [w566 w576] -> w525
                  tunnel: w526 -> [w553 _]
                  tunnel: w524 -> [_ w576]
                  tunnel: w520 -> [_ _]
                  tunnel: w519 -> [w544 _]
                  tunnel: w518 -> [w542 _]
                  tunnel: w517 -> [w539 _]
                  frame False {
                    # "dt = t2 -t1"
                    n186 = call "GetTimeInSeconds.vi"("Timestamp"=w553) -> ("Numeric"=w547:dbl)  [unwired: 10 in]
                    n187 = feedback-in #23(w547) -> ()
                    n188 = feedback #23(0.0 ("Numeric")) -> (w546:dbl)
                    n189 = Index Array(array=w540) -> (element #1=w555:dbl[], element #2=w558:dbl[])  [unwired: 4 in]
                    n190 = Subtract(x=w547, y=w546) -> (x-y=w549:dbl)
                    n191 = Empty Array?(array=w555) -> (empty?=w556:bool)
                    n192 = feedback #24(0.015 ("Numeric")) -> (w548:dbl)
                    n193 = Select(t=w567, s=w556, f=w555) -> (s? t:f=w554:dbl[])
                    n194 = Empty Array?(array=w558) -> (empty?=w559:bool)
                    n195 = Equal?(x=w549, y=0.0) -> (x = y?=w552:bool)
                    n196 = Select(t=w554, s=w559, f=w558) -> (s? t:f=w557:dbl[])
                    n197 = Select(t=w548, s=w552, f=w549) -> (s? t:f=w543:dbl)
                    n198 = call "PathVelocityProfile.vi"("Pose"=w567, "time"=w547, "intervalo"=w543, "estimatives"=w569, "Path  Smooth"=w540, "V_max"=w575, "Accel"=w574, "DesAccel"=w573) -> ("Time X"=w565:dbl[], "Velocities X"=w564:dbl[], "Time Y"=w563:dbl[], "Velocities Y"=w562:dbl[])  [unwired: 4 in]
                    n199 = call "VelocityCommand.vi"("intervalo"=w543, "MaxOutputXY"=w542, "estimatives"=w569, "Velocities Y"=w562, "Time Y"=w563, "Velocities X"=w564, "Time X"=w565) -> ("Vy"=w561:dbl, "Vx"=w560:dbl)  [unwired: 3 in]
                    n200 = feedback-in #24(w543) -> ()
                    n201 = call "VelocityControl.vi"("estimatives"=w569, "Dest_orientation"=w568, "Position"=w567, "Waypoint 1"=w557, "Waypoint 0"=w554, "Vx"=w560, "Project"=Project."VSS", "Vy"=w561, "VSSStates"=w539, "output xy"=w570, "output inc"=w572, "output angle"=w571, "PID gains Vel"=w544, "Path  Smooth"=w540) -> ("Output Velocity"=w566:dbl[])  [unwired: 1 in]
                  }
                  frame True {
                  }
                }
                n202 = feedback-in #22(w525) -> ()
                n203 = Index Array(array=w524) -> (element #1=w529:dbl, element #2=w528:dbl, element #3=w527:dbl)  [unwired: 3 in]
              }
              frame 8 {
                n204 = Not A Number/Path/Refnum?(number/path/refnum=w583) -> (NaN/Path/Refnum?=w582:bool[][])
                n205 = Or Array Elements(Boolean array=w582) -> (logical OR=w581:bool)
                n206 = feedback #25() -> (w584:dbl[])  [unwired: 1 in]
                n207 = case shown="False" w581 {
                  tunnel: w598 -> [w635 _]
                  tunnel: w597 -> [w634 _]
                  tunnel: w596 -> [w633 _]
                  tunnel: w595 -> [w632 _]
                  tunnel: w594 -> [w631 _]
                  tunnel: w593 -> [w630 _]
                  tunnel: w592 -> [w629 _]
                  tunnel: w591 -> [w628 _]
                  tunnel: w583 -> [w600 _]
                  tunnel: w590 -> [w627 _]
                  tunnel: [w626 w636] -> w585
                  tunnel: w586 -> [w613 _]
                  tunnel: w584 -> [_ w636]
                  tunnel: w580 -> [_ _]
                  tunnel: w579 -> [w604 _]
                  tunnel: w578 -> [w602 _]
                  tunnel: w577 -> [w599 _]
                  frame False {
                    # "dt = t2 -t1"
                    n208 = call "GetTimeInSeconds.vi"("Timestamp"=w613) -> ("Numeric"=w607:dbl)  [unwired: 10 in]
                    n209 = feedback-in #26(w607) -> ()
                    n210 = feedback #26(0.0 ("Numeric")) -> (w606:dbl)
                    n211 = Index Array(array=w600) -> (element #1=w615:dbl[], element #2=w618:dbl[])  [unwired: 4 in]
                    n212 = Subtract(x=w607, y=w606) -> (x-y=w609:dbl)
                    n213 = Empty Array?(array=w615) -> (empty?=w616:bool)
                    n214 = feedback #27(0.015 ("Numeric")) -> (w608:dbl)
                    n215 = Select(t=w627, s=w616, f=w615) -> (s? t:f=w614:dbl[])
                    n216 = Empty Array?(array=w618) -> (empty?=w619:bool)
                    n217 = Equal?(x=w609, y=0.0) -> (x = y?=w612:bool)
                    n218 = Select(t=w614, s=w619, f=w618) -> (s? t:f=w617:dbl[])
                    n219 = Select(t=w608, s=w612, f=w609) -> (s? t:f=w603:dbl)
                    n220 = call "PathVelocityProfile.vi"("Pose"=w627, "time"=w607, "intervalo"=w603, "estimatives"=w629, "Path  Smooth"=w600, "V_max"=w635, "Accel"=w634, "DesAccel"=w633) -> ("Time X"=w625:dbl[], "Velocities X"=w624:dbl[], "Time Y"=w623:dbl[], "Velocities Y"=w622:dbl[])  [unwired: 4 in]
                    n221 = call "VelocityCommand.vi"("intervalo"=w603, "MaxOutputXY"=w602, "estimatives"=w629, "Velocities Y"=w622, "Time Y"=w623, "Velocities X"=w624, "Time X"=w625) -> ("Vy"=w621:dbl, "Vx"=w620:dbl)  [unwired: 3 in]
                    n222 = feedback-in #27(w603) -> ()
                    n223 = call "VelocityControl.vi"("estimatives"=w629, "Dest_orientation"=w628, "Position"=w627, "Waypoint 1"=w617, "Waypoint 0"=w614, "Vx"=w620, "Project"=Project."VSS", "Vy"=w621, "VSSStates"=w599, "output xy"=w630, "output inc"=w632, "output angle"=w631, "PID gains Vel"=w604, "Path  Smooth"=w600) -> ("Output Velocity"=w626:dbl[])  [unwired: 1 in]
                  }
                  frame True {
                  }
                }
                n224 = feedback-in #25(w585) -> ()
                n225 = Index Array(array=w584) -> (element #1=w589:dbl, element #2=w588:dbl, element #3=w587:dbl)  [unwired: 3 in]
              }
              frame 9 {
                n226 = Not A Number/Path/Refnum?(number/path/refnum=w643) -> (NaN/Path/Refnum?=w642:bool[][])
                n227 = Or Array Elements(Boolean array=w642) -> (logical OR=w641:bool)
                n228 = feedback #28() -> (w644:dbl[])  [unwired: 1 in]
                n229 = case shown="False" w641 {
                  tunnel: w658 -> [w695 _]
                  tunnel: w657 -> [w694 _]
                  tunnel: w656 -> [w693 _]
                  tunnel: w655 -> [w692 _]
                  tunnel: w654 -> [w691 _]
                  tunnel: w653 -> [w690 _]
                  tunnel: w652 -> [w689 _]
                  tunnel: w651 -> [w688 _]
                  tunnel: w643 -> [w660 _]
                  tunnel: w650 -> [w687 _]
                  tunnel: [w686 w696] -> w645
                  tunnel: w646 -> [w673 _]
                  tunnel: w644 -> [_ w696]
                  tunnel: w640 -> [_ _]
                  tunnel: w639 -> [w664 _]
                  tunnel: w638 -> [w662 _]
                  tunnel: w637 -> [w659 _]
                  frame False {
                    # "dt = t2 -t1"
                    n230 = call "GetTimeInSeconds.vi"("Timestamp"=w673) -> ("Numeric"=w667:dbl)  [unwired: 10 in]
                    n231 = feedback-in #29(w667) -> ()
                    n232 = feedback #29(0.0 ("Numeric")) -> (w666:dbl)
                    n233 = Index Array(array=w660) -> (element #1=w675:dbl[], element #2=w678:dbl[])  [unwired: 4 in]
                    n234 = Subtract(x=w667, y=w666) -> (x-y=w669:dbl)
                    n235 = Empty Array?(array=w675) -> (empty?=w676:bool)
                    n236 = feedback #30(0.015 ("Numeric")) -> (w668:dbl)
                    n237 = Select(t=w687, s=w676, f=w675) -> (s? t:f=w674:dbl[])
                    n238 = Empty Array?(array=w678) -> (empty?=w679:bool)
                    n239 = Equal?(x=w669, y=0.0) -> (x = y?=w672:bool)
                    n240 = Select(t=w674, s=w679, f=w678) -> (s? t:f=w677:dbl[])
                    n241 = Select(t=w668, s=w672, f=w669) -> (s? t:f=w663:dbl)
                    n242 = call "PathVelocityProfile.vi"("Pose"=w687, "time"=w667, "intervalo"=w663, "estimatives"=w689, "Path  Smooth"=w660, "V_max"=w695, "Accel"=w694, "DesAccel"=w693) -> ("Time X"=w685:dbl[], "Velocities X"=w684:dbl[], "Time Y"=w683:dbl[], "Velocities Y"=w682:dbl[])  [unwired: 4 in]
                    n243 = call "VelocityCommand.vi"("intervalo"=w663, "MaxOutputXY"=w662, "estimatives"=w689, "Velocities Y"=w682, "Time Y"=w683, "Velocities X"=w684, "Time X"=w685) -> ("Vy"=w681:dbl, "Vx"=w680:dbl)  [unwired: 3 in]
                    n244 = feedback-in #30(w663) -> ()
                    n245 = call "VelocityControl.vi"("estimatives"=w689, "Dest_orientation"=w688, "Position"=w687, "Waypoint 1"=w677, "Waypoint 0"=w674, "Vx"=w680, "Project"=Project."VSS", "Vy"=w681, "VSSStates"=w659, "output xy"=w690, "output inc"=w692, "output angle"=w691, "PID gains Vel"=w664, "Path  Smooth"=w660) -> ("Output Velocity"=w686:dbl[])  [unwired: 1 in]
                  }
                  frame True {
                  }
                }
                n246 = feedback-in #28(w645) -> ()
                n247 = Index Array(array=w644) -> (element #1=w649:dbl, element #2=w648:dbl, element #3=w647:dbl)  [unwired: 3 in]
              }
              frame 10 {
                n248 = Not A Number/Path/Refnum?(number/path/refnum=w703) -> (NaN/Path/Refnum?=w702:bool[][])
                n249 = Or Array Elements(Boolean array=w702) -> (logical OR=w701:bool)
                n250 = feedback #31() -> (w704:dbl[])  [unwired: 1 in]
                n251 = case shown="False" w701 {
                  tunnel: w718 -> [w755 _]
                  tunnel: w717 -> [w754 _]
                  tunnel: w716 -> [w753 _]
                  tunnel: w715 -> [w752 _]
                  tunnel: w714 -> [w751 _]
                  tunnel: w713 -> [w750 _]
                  tunnel: w712 -> [w749 _]
                  tunnel: w711 -> [w748 _]
                  tunnel: w703 -> [w720 _]
                  tunnel: w710 -> [w747 _]
                  tunnel: [w746 w756] -> w705
                  tunnel: w706 -> [w733 _]
                  tunnel: w704 -> [_ w756]
                  tunnel: w700 -> [_ _]
                  tunnel: w699 -> [w724 _]
                  tunnel: w698 -> [w722 _]
                  tunnel: w697 -> [w719 _]
                  frame False {
                    # "dt = t2 -t1"
                    n252 = call "GetTimeInSeconds.vi"("Timestamp"=w733) -> ("Numeric"=w727:dbl)  [unwired: 10 in]
                    n253 = feedback-in #32(w727) -> ()
                    n254 = feedback #32(0.0 ("Numeric")) -> (w726:dbl)
                    n255 = Index Array(array=w720) -> (element #1=w735:dbl[], element #2=w738:dbl[])  [unwired: 4 in]
                    n256 = Subtract(x=w727, y=w726) -> (x-y=w729:dbl)
                    n257 = Empty Array?(array=w735) -> (empty?=w736:bool)
                    n258 = feedback #33(0.015 ("Numeric")) -> (w728:dbl)
                    n259 = Select(t=w747, s=w736, f=w735) -> (s? t:f=w734:dbl[])
                    n260 = Empty Array?(array=w738) -> (empty?=w739:bool)
                    n261 = Equal?(x=w729, y=0.0) -> (x = y?=w732:bool)
                    n262 = Select(t=w734, s=w739, f=w738) -> (s? t:f=w737:dbl[])
                    n263 = Select(t=w728, s=w732, f=w729) -> (s? t:f=w723:dbl)
                    n264 = call "PathVelocityProfile.vi"("Pose"=w747, "time"=w727, "intervalo"=w723, "estimatives"=w749, "Path  Smooth"=w720, "V_max"=w755, "Accel"=w754, "DesAccel"=w753) -> ("Time X"=w745:dbl[], "Velocities X"=w744:dbl[], "Time Y"=w743:dbl[], "Velocities Y"=w742:dbl[])  [unwired: 4 in]
                    n265 = call "VelocityCommand.vi"("intervalo"=w723, "MaxOutputXY"=w722, "estimatives"=w749, "Velocities Y"=w742, "Time Y"=w743, "Velocities X"=w744, "Time X"=w745) -> ("Vy"=w741:dbl, "Vx"=w740:dbl)  [unwired: 3 in]
                    n266 = feedback-in #33(w723) -> ()
                    n267 = call "VelocityControl.vi"("estimatives"=w749, "Dest_orientation"=w748, "Position"=w747, "Waypoint 1"=w737, "Waypoint 0"=w734, "Vx"=w740, "Project"=Project."VSS", "Vy"=w741, "VSSStates"=w719, "output xy"=w750, "output inc"=w752, "output angle"=w751, "PID gains Vel"=w724, "Path  Smooth"=w720) -> ("Output Velocity"=w746:dbl[])  [unwired: 1 in]
                  }
                  frame True {
                  }
                }
                n268 = feedback-in #31(w705) -> ()
                n269 = Index Array(array=w704) -> (element #1=w709:dbl, element #2=w708:dbl, element #3=w707:dbl)  [unwired: 3 in]
              }
              frame 11 {
                n270 = Not A Number/Path/Refnum?(number/path/refnum=w763) -> (NaN/Path/Refnum?=w762:bool[][])
                n271 = Or Array Elements(Boolean array=w762) -> (logical OR=w761:bool)
                n272 = feedback #34() -> (w764:dbl[])  [unwired: 1 in]
                n273 = case shown="False" w761 {
                  tunnel: w778 -> [w815 _]
                  tunnel: w777 -> [w814 _]
                  tunnel: w776 -> [w813 _]
                  tunnel: w775 -> [w812 _]
                  tunnel: w774 -> [w811 _]
                  tunnel: w773 -> [w810 _]
                  tunnel: w772 -> [w809 _]
                  tunnel: w771 -> [w808 _]
                  tunnel: w763 -> [w780 _]
                  tunnel: w770 -> [w807 _]
                  tunnel: [w806 w816] -> w765
                  tunnel: w766 -> [w793 _]
                  tunnel: w764 -> [_ w816]
                  tunnel: w760 -> [_ _]
                  tunnel: w759 -> [w784 _]
                  tunnel: w758 -> [w782 _]
                  tunnel: w757 -> [w779 _]
                  frame False {
                    # "dt = t2 -t1"
                    n274 = call "GetTimeInSeconds.vi"("Timestamp"=w793) -> ("Numeric"=w787:dbl)  [unwired: 10 in]
                    n275 = feedback-in #35(w787) -> ()
                    n276 = feedback #35(0.0 ("Numeric")) -> (w786:dbl)
                    n277 = Index Array(array=w780) -> (element #1=w795:dbl[], element #2=w798:dbl[])  [unwired: 4 in]
                    n278 = Subtract(x=w787, y=w786) -> (x-y=w789:dbl)
                    n279 = Empty Array?(array=w795) -> (empty?=w796:bool)
                    n280 = feedback #36(0.015 ("Numeric")) -> (w788:dbl)
                    n281 = Select(t=w807, s=w796, f=w795) -> (s? t:f=w794:dbl[])
                    n282 = Empty Array?(array=w798) -> (empty?=w799:bool)
                    n283 = Equal?(x=w789, y=0.0) -> (x = y?=w792:bool)
                    n284 = Select(t=w794, s=w799, f=w798) -> (s? t:f=w797:dbl[])
                    n285 = Select(t=w788, s=w792, f=w789) -> (s? t:f=w783:dbl)
                    n286 = call "PathVelocityProfile.vi"("Pose"=w807, "time"=w787, "intervalo"=w783, "estimatives"=w809, "Path  Smooth"=w780, "V_max"=w815, "Accel"=w814, "DesAccel"=w813) -> ("Time X"=w805:dbl[], "Velocities X"=w804:dbl[], "Time Y"=w803:dbl[], "Velocities Y"=w802:dbl[])  [unwired: 4 in]
                    n287 = call "VelocityCommand.vi"("intervalo"=w783, "MaxOutputXY"=w782, "estimatives"=w809, "Velocities Y"=w802, "Time Y"=w803, "Velocities X"=w804, "Time X"=w805) -> ("Vy"=w801:dbl, "Vx"=w800:dbl)  [unwired: 3 in]
                    n288 = feedback-in #36(w783) -> ()
                    n289 = call "VelocityControl.vi"("estimatives"=w809, "Dest_orientation"=w808, "Position"=w807, "Waypoint 1"=w797, "Waypoint 0"=w794, "Vx"=w800, "Project"=Project."VSS", "Vy"=w801, "VSSStates"=w779, "output xy"=w810, "output inc"=w812, "output angle"=w811, "PID gains Vel"=w784, "Path  Smooth"=w780) -> ("Output Velocity"=w806:dbl[])  [unwired: 1 in]
                  }
                  frame True {
                  }
                }
                n290 = feedback-in #34(w765) -> ()
                n291 = Index Array(array=w764) -> (element #1=w769:dbl, element #2=w768:dbl, element #3=w767:dbl)  [unwired: 3 in]
              }
              frame 12 {
                n292 = Not A Number/Path/Refnum?(number/path/refnum=w823) -> (NaN/Path/Refnum?=w822:bool[][])
                n293 = Or Array Elements(Boolean array=w822) -> (logical OR=w821:bool)
                n294 = feedback #37() -> (w824:dbl[])  [unwired: 1 in]
                n295 = case shown="False" w821 {
                  tunnel: w838 -> [w875 _]
                  tunnel: w837 -> [w874 _]
                  tunnel: w836 -> [w873 _]
                  tunnel: w835 -> [w872 _]
                  tunnel: w834 -> [w871 _]
                  tunnel: w833 -> [w870 _]
                  tunnel: w832 -> [w869 _]
                  tunnel: w831 -> [w868 _]
                  tunnel: w823 -> [w840 _]
                  tunnel: w830 -> [w867 _]
                  tunnel: [w866 w876] -> w825
                  tunnel: w826 -> [w853 _]
                  tunnel: w824 -> [_ w876]
                  tunnel: w820 -> [_ _]
                  tunnel: w819 -> [w844 _]
                  tunnel: w818 -> [w842 _]
                  tunnel: w817 -> [w839 _]
                  frame False {
                    # "dt = t2 -t1"
                    n296 = call "GetTimeInSeconds.vi"("Timestamp"=w853) -> ("Numeric"=w847:dbl)  [unwired: 10 in]
                    n297 = feedback-in #38(w847) -> ()
                    n298 = feedback #38(0.0 ("Numeric")) -> (w846:dbl)
                    n299 = Index Array(array=w840) -> (element #1=w855:dbl[], element #2=w858:dbl[])  [unwired: 4 in]
                    n300 = Subtract(x=w847, y=w846) -> (x-y=w849:dbl)
                    n301 = Empty Array?(array=w855) -> (empty?=w856:bool)
                    n302 = feedback #39(0.015 ("Numeric")) -> (w848:dbl)
                    n303 = Select(t=w867, s=w856, f=w855) -> (s? t:f=w854:dbl[])
                    n304 = Empty Array?(array=w858) -> (empty?=w859:bool)
                    n305 = Equal?(x=w849, y=0.0) -> (x = y?=w852:bool)
                    n306 = Select(t=w854, s=w859, f=w858) -> (s? t:f=w857:dbl[])
                    n307 = Select(t=w848, s=w852, f=w849) -> (s? t:f=w843:dbl)
                    n308 = call "PathVelocityProfile.vi"("Pose"=w867, "time"=w847, "intervalo"=w843, "estimatives"=w869, "Path  Smooth"=w840, "V_max"=w875, "Accel"=w874, "DesAccel"=w873) -> ("Time X"=w865:dbl[], "Velocities X"=w864:dbl[], "Time Y"=w863:dbl[], "Velocities Y"=w862:dbl[])  [unwired: 4 in]
                    n309 = call "VelocityCommand.vi"("intervalo"=w843, "MaxOutputXY"=w842, "estimatives"=w869, "Velocities Y"=w862, "Time Y"=w863, "Velocities X"=w864, "Time X"=w865) -> ("Vy"=w861:dbl, "Vx"=w860:dbl)  [unwired: 3 in]
                    n310 = feedback-in #39(w843) -> ()
                    n311 = call "VelocityControl.vi"("estimatives"=w869, "Dest_orientation"=w868, "Position"=w867, "Waypoint 1"=w857, "Waypoint 0"=w854, "Vx"=w860, "Project"=Project."VSS", "Vy"=w861, "VSSStates"=w839, "output xy"=w870, "output inc"=w872, "output angle"=w871, "PID gains Vel"=w844, "Path  Smooth"=w840) -> ("Output Velocity"=w866:dbl[])  [unwired: 1 in]
                  }
                  frame True {
                  }
                }
                n312 = feedback-in #37(w825) -> ()
                n313 = Index Array(array=w824) -> (element #1=w829:dbl, element #2=w828:dbl, element #3=w827:dbl)  [unwired: 3 in]
              }
              frame 13 {
                n314 = Not A Number/Path/Refnum?(number/path/refnum=w883) -> (NaN/Path/Refnum?=w882:bool[][])
                n315 = Or Array Elements(Boolean array=w882) -> (logical OR=w881:bool)
                n316 = feedback #40() -> (w884:dbl[])  [unwired: 1 in]
                n317 = case shown="False" w881 {
                  tunnel: w898 -> [w935 _]
                  tunnel: w897 -> [w934 _]
                  tunnel: w896 -> [w933 _]
                  tunnel: w895 -> [w932 _]
                  tunnel: w894 -> [w931 _]
                  tunnel: w893 -> [w930 _]
                  tunnel: w892 -> [w929 _]
                  tunnel: w891 -> [w928 _]
                  tunnel: w883 -> [w900 _]
                  tunnel: w890 -> [w927 _]
                  tunnel: [w926 w936] -> w885
                  tunnel: w886 -> [w913 _]
                  tunnel: w884 -> [_ w936]
                  tunnel: w880 -> [_ _]
                  tunnel: w879 -> [w904 _]
                  tunnel: w878 -> [w902 _]
                  tunnel: w877 -> [w899 _]
                  frame False {
                    # "dt = t2 -t1"
                    n318 = call "GetTimeInSeconds.vi"("Timestamp"=w913) -> ("Numeric"=w907:dbl)  [unwired: 10 in]
                    n319 = feedback-in #41(w907) -> ()
                    n320 = feedback #41(0.0 ("Numeric")) -> (w906:dbl)
                    n321 = Index Array(array=w900) -> (element #1=w915:dbl[], element #2=w918:dbl[])  [unwired: 4 in]
                    n322 = Subtract(x=w907, y=w906) -> (x-y=w909:dbl)
                    n323 = Empty Array?(array=w915) -> (empty?=w916:bool)
                    n324 = feedback #42(0.015 ("Numeric")) -> (w908:dbl)
                    n325 = Select(t=w927, s=w916, f=w915) -> (s? t:f=w914:dbl[])
                    n326 = Empty Array?(array=w918) -> (empty?=w919:bool)
                    n327 = Equal?(x=w909, y=0.0) -> (x = y?=w912:bool)
                    n328 = Select(t=w914, s=w919, f=w918) -> (s? t:f=w917:dbl[])
                    n329 = Select(t=w908, s=w912, f=w909) -> (s? t:f=w903:dbl)
                    n330 = call "PathVelocityProfile.vi"("Pose"=w927, "time"=w907, "intervalo"=w903, "estimatives"=w929, "Path  Smooth"=w900, "V_max"=w935, "Accel"=w934, "DesAccel"=w933) -> ("Time X"=w925:dbl[], "Velocities X"=w924:dbl[], "Time Y"=w923:dbl[], "Velocities Y"=w922:dbl[])  [unwired: 4 in]
                    n331 = call "VelocityCommand.vi"("intervalo"=w903, "MaxOutputXY"=w902, "estimatives"=w929, "Velocities Y"=w922, "Time Y"=w923, "Velocities X"=w924, "Time X"=w925) -> ("Vy"=w921:dbl, "Vx"=w920:dbl)  [unwired: 3 in]
                    n332 = feedback-in #42(w903) -> ()
                    n333 = call "VelocityControl.vi"("estimatives"=w929, "Dest_orientation"=w928, "Position"=w927, "Waypoint 1"=w917, "Waypoint 0"=w914, "Vx"=w920, "Project"=Project."VSS", "Vy"=w921, "VSSStates"=w899, "output xy"=w930, "output inc"=w932, "output angle"=w931, "PID gains Vel"=w904, "Path  Smooth"=w900) -> ("Output Velocity"=w926:dbl[])  [unwired: 1 in]
                  }
                  frame True {
                  }
                }
                n334 = feedback-in #40(w885) -> ()
                n335 = Index Array(array=w884) -> (element #1=w889:dbl, element #2=w888:dbl, element #3=w887:dbl)  [unwired: 3 in]
              }
              frame 14 {
                n336 = Not A Number/Path/Refnum?(number/path/refnum=w943) -> (NaN/Path/Refnum?=w942:bool[][])
                n337 = Or Array Elements(Boolean array=w942) -> (logical OR=w941:bool)
                n338 = feedback #43() -> (w944:dbl[])  [unwired: 1 in]
                n339 = case shown="False" w941 {
                  tunnel: w958 -> [w995 _]
                  tunnel: w957 -> [w994 _]
                  tunnel: w956 -> [w993 _]
                  tunnel: w955 -> [w992 _]
                  tunnel: w954 -> [w991 _]
                  tunnel: w953 -> [w990 _]
                  tunnel: w952 -> [w989 _]
                  tunnel: w951 -> [w988 _]
                  tunnel: w943 -> [w960 _]
                  tunnel: w950 -> [w987 _]
                  tunnel: [w986 w996] -> w945
                  tunnel: w946 -> [w973 _]
                  tunnel: w944 -> [_ w996]
                  tunnel: w940 -> [_ _]
                  tunnel: w939 -> [w964 _]
                  tunnel: w938 -> [w962 _]
                  tunnel: w937 -> [w959 _]
                  frame False {
                    # "dt = t2 -t1"
                    n340 = call "GetTimeInSeconds.vi"("Timestamp"=w973) -> ("Numeric"=w967:dbl)  [unwired: 10 in]
                    n341 = feedback-in #44(w967) -> ()
                    n342 = feedback #44(0.0 ("Numeric")) -> (w966:dbl)
                    n343 = Index Array(array=w960) -> (element #1=w975:dbl[], element #2=w978:dbl[])  [unwired: 4 in]
                    n344 = Subtract(x=w967, y=w966) -> (x-y=w969:dbl)
                    n345 = Empty Array?(array=w975) -> (empty?=w976:bool)
                    n346 = feedback #45(0.015 ("Numeric")) -> (w968:dbl)
                    n347 = Select(t=w987, s=w976, f=w975) -> (s? t:f=w974:dbl[])
                    n348 = Empty Array?(array=w978) -> (empty?=w979:bool)
                    n349 = Equal?(x=w969, y=0.0) -> (x = y?=w972:bool)
                    n350 = Select(t=w974, s=w979, f=w978) -> (s? t:f=w977:dbl[])
                    n351 = Select(t=w968, s=w972, f=w969) -> (s? t:f=w963:dbl)
                    n352 = call "PathVelocityProfile.vi"("Pose"=w987, "time"=w967, "intervalo"=w963, "estimatives"=w989, "Path  Smooth"=w960, "V_max"=w995, "Accel"=w994, "DesAccel"=w993) -> ("Time X"=w985:dbl[], "Velocities X"=w984:dbl[], "Time Y"=w983:dbl[], "Velocities Y"=w982:dbl[])  [unwired: 4 in]
                    n353 = call "VelocityCommand.vi"("intervalo"=w963, "MaxOutputXY"=w962, "estimatives"=w989, "Velocities Y"=w982, "Time Y"=w983, "Velocities X"=w984, "Time X"=w985) -> ("Vy"=w981:dbl, "Vx"=w980:dbl)  [unwired: 3 in]
                    n354 = feedback-in #45(w963) -> ()
                    n355 = call "VelocityControl.vi"("estimatives"=w989, "Dest_orientation"=w988, "Position"=w987, "Waypoint 1"=w977, "Waypoint 0"=w974, "Vx"=w980, "Project"=Project."VSS", "Vy"=w981, "VSSStates"=w959, "output xy"=w990, "output inc"=w992, "output angle"=w991, "PID gains Vel"=w964, "Path  Smooth"=w960) -> ("Output Velocity"=w986:dbl[])  [unwired: 1 in]
                  }
                  frame True {
                  }
                }
                n356 = feedback-in #43(w945) -> ()
                n357 = Index Array(array=w944) -> (element #1=w949:dbl, element #2=w948:dbl, element #3=w947:dbl)  [unwired: 3 in]
              }
              frame 15 {
                n358 = Not A Number/Path/Refnum?(number/path/refnum=w1003) -> (NaN/Path/Refnum?=w1002:bool[][])
                n359 = Or Array Elements(Boolean array=w1002) -> (logical OR=w1001:bool)
                n360 = feedback #46() -> (w1004:dbl[])  [unwired: 1 in]
                n361 = case shown="False" w1001 {
                  tunnel: w1018 -> [w1055 _]
                  tunnel: w1017 -> [w1054 _]
                  tunnel: w1016 -> [w1053 _]
                  tunnel: w1015 -> [w1052 _]
                  tunnel: w1014 -> [w1051 _]
                  tunnel: w1013 -> [w1050 _]
                  tunnel: w1012 -> [w1049 _]
                  tunnel: w1011 -> [w1048 _]
                  tunnel: w1003 -> [w1020 _]
                  tunnel: w1010 -> [w1047 _]
                  tunnel: [w1046 w1056] -> w1005
                  tunnel: w1006 -> [w1033 _]
                  tunnel: w1004 -> [_ w1056]
                  tunnel: w1000 -> [_ _]
                  tunnel: w999 -> [w1024 _]
                  tunnel: w998 -> [w1022 _]
                  tunnel: w997 -> [w1019 _]
                  frame False {
                    # "dt = t2 -t1"
                    n362 = call "GetTimeInSeconds.vi"("Timestamp"=w1033) -> ("Numeric"=w1027:dbl)  [unwired: 10 in]
                    n363 = feedback-in #47(w1027) -> ()
                    n364 = feedback #47(0.0 ("Numeric")) -> (w1026:dbl)
                    n365 = Index Array(array=w1020) -> (element #1=w1035:dbl[], element #2=w1038:dbl[])  [unwired: 4 in]
                    n366 = Subtract(x=w1027, y=w1026) -> (x-y=w1029:dbl)
                    n367 = Empty Array?(array=w1035) -> (empty?=w1036:bool)
                    n368 = feedback #48(0.015 ("Numeric")) -> (w1028:dbl)
                    n369 = Select(t=w1047, s=w1036, f=w1035) -> (s? t:f=w1034:dbl[])
                    n370 = Empty Array?(array=w1038) -> (empty?=w1039:bool)
                    n371 = Equal?(x=w1029, y=0.0) -> (x = y?=w1032:bool)
                    n372 = Select(t=w1034, s=w1039, f=w1038) -> (s? t:f=w1037:dbl[])
                    n373 = Select(t=w1028, s=w1032, f=w1029) -> (s? t:f=w1023:dbl)
                    n374 = call "PathVelocityProfile.vi"("Pose"=w1047, "time"=w1027, "intervalo"=w1023, "estimatives"=w1049, "Path  Smooth"=w1020, "V_max"=w1055, "Accel"=w1054, "DesAccel"=w1053) -> ("Time X"=w1045:dbl[], "Velocities X"=w1044:dbl[], "Time Y"=w1043:dbl[], "Velocities Y"=w1042:dbl[])  [unwired: 4 in]
                    n375 = call "VelocityCommand.vi"("intervalo"=w1023, "MaxOutputXY"=w1022, "estimatives"=w1049, "Velocities Y"=w1042, "Time Y"=w1043, "Velocities X"=w1044, "Time X"=w1045) -> ("Vy"=w1041:dbl, "Vx"=w1040:dbl)  [unwired: 3 in]
                    n376 = feedback-in #48(w1023) -> ()
                    n377 = call "VelocityControl.vi"("estimatives"=w1049, "Dest_orientation"=w1048, "Position"=w1047, "Waypoint 1"=w1037, "Waypoint 0"=w1034, "Vx"=w1040, "Project"=Project."VSS", "Vy"=w1041, "VSSStates"=w1019, "output xy"=w1050, "output inc"=w1052, "output angle"=w1051, "PID gains Vel"=w1024, "Path  Smooth"=w1020) -> ("Output Velocity"=w1046:dbl[])  [unwired: 1 in]
                  }
                  frame True {
                  }
                }
                n378 = feedback-in #46(w1005) -> ()
                n379 = Index Array(array=w1004) -> (element #1=w1009:dbl, element #2=w1008:dbl, element #3=w1007:dbl)  [unwired: 3 in]
              }
            }
          }
          frame True {
            w1057 = 0.0 ("output")
          }
        }
        n380 = Bundle By Name(cluster=w77, "v_tangent"=w62, "v_normal"=w61, "v_ang"=w57) -> (w76:T3)
      }
      n381 = Bundle By Name(cluster=w35, "our_robots"=w36) -> (w34:T2)
    }
    frame True {
      n382 = for {
        tunnel: w1062 -> [w1078] mode=indexing
        tunnel: w1061 -> [w1084]
        tunnel: [w1075] -> w1058 mode=indexing
        # "v_tangent = v_left\nv_normal = v_rigth"
        n383 = Unbundle By Name(w1078) -> ("id"=w1074:u32, "x"=w1083:dbl, "y"=w1082:dbl, "orientation"=w1081:dbl, "Path  Smooth"=w1079:dbl[][], "VSSStates"=w1073:T8)
        n384 = Build Array(w1083, w1082, w1081) -> (w1080:dbl[])
        n385 = Negate(x=0.15 ("upper limit")) -> (-x=w1070:dbl)
        n386 = Negate(x=0.15 ("upper limit")) -> (-x=w1069:dbl)
        n387 = case shown="0, Default" w1074 {
          selector: w1074 -> [w1085 w1091 w1097 w1103 w1109 w1115 w1121 w1127 w1133 w1139 w1145 w1151 w1157 w1163 w1169 w1175]
          tunnel: w1084 -> [w1090 w1096 w1102 w1108 w1114 w1120 w1126 w1132 w1138 w1144 w1150 w1156 w1162 w1168 w1174 w1180]
          tunnel: w1080 -> [w1089 w1095 w1101 w1107 w1113 w1119 w1125 w1131 w1137 w1143 w1149 w1155 w1161 w1167 w1173 w1179]
          tunnel: w1079 -> [w1088 w1094 w1100 w1106 w1112 w1118 w1124 w1130 w1136 w1142 w1148 w1154 w1160 w1166 w1172 w1178]
          tunnel: [w1087 w1093 w1099 w1105 w1111 w1117 w1123 w1129 w1135 w1141 w1147 w1153 w1159 w1165 w1171 w1177] -> w1077
          tunnel: w1073 -> [w1086 w1092 w1098 w1104 w1110 w1116 w1122 w1128 w1134 w1140 w1146 w1152 w1158 w1164 w1170 w1176]
          frame 0, Default {
            n388 = call "NewVSS_GoTo.vi"("VSSStates"=w1086, "Numeric"=w1085, "Path  Smooth"=w1088, "Position"=w1089, "GoToNavigation?"=w1090) -> ("Output Velocity"=w1087:dbl[])  [unwired: 6 in]
          }
          frame 1 {
            n389 = call "NewVSS_GoTo.vi"("VSSStates"=w1092, "Numeric"=w1091, "Path  Smooth"=w1094, "Position"=w1095, "GoToNavigation?"=w1096) -> ("Output Velocity"=w1093:dbl[])  [unwired: 6 in]
          }
          frame 2 {
            n390 = call "NewVSS_GoTo.vi"("VSSStates"=w1098, "Numeric"=w1097, "Path  Smooth"=w1100, "Position"=w1101, "GoToNavigation?"=w1102) -> ("Output Velocity"=w1099:dbl[])  [unwired: 6 in]
          }
          frame 3 {
            n391 = call "NewVSS_GoTo.vi"("VSSStates"=w1104, "Numeric"=w1103, "Path  Smooth"=w1106, "Position"=w1107, "GoToNavigation?"=w1108) -> ("Output Velocity"=w1105:dbl[])  [unwired: 6 in]
          }
          frame 4 {
            n392 = call "NewVSS_GoTo.vi"("VSSStates"=w1110, "Numeric"=w1109, "Path  Smooth"=w1112, "Position"=w1113, "GoToNavigation?"=w1114) -> ("Output Velocity"=w1111:dbl[])  [unwired: 6 in]
          }
          frame 5 {
            n393 = call "NewVSS_GoTo.vi"("VSSStates"=w1116, "Numeric"=w1115, "Path  Smooth"=w1118, "Position"=w1119, "GoToNavigation?"=w1120) -> ("Output Velocity"=w1117:dbl[])  [unwired: 6 in]
          }
          frame 6 {
            n394 = call "NewVSS_GoTo.vi"("VSSStates"=w1122, "Numeric"=w1121, "Path  Smooth"=w1124, "Position"=w1125, "GoToNavigation?"=w1126) -> ("Output Velocity"=w1123:dbl[])  [unwired: 6 in]
          }
          frame 7 {
            n395 = call "NewVSS_GoTo.vi"("VSSStates"=w1128, "Numeric"=w1127, "Path  Smooth"=w1130, "Position"=w1131, "GoToNavigation?"=w1132) -> ("Output Velocity"=w1129:dbl[])  [unwired: 6 in]
          }
          frame 8 {
            n396 = call "NewVSS_GoTo.vi"("VSSStates"=w1134, "Numeric"=w1133, "Path  Smooth"=w1136, "Position"=w1137, "GoToNavigation?"=w1138) -> ("Output Velocity"=w1135:dbl[])  [unwired: 6 in]
          }
          frame 9 {
            n397 = call "NewVSS_GoTo.vi"("VSSStates"=w1140, "Numeric"=w1139, "Path  Smooth"=w1142, "Position"=w1143, "GoToNavigation?"=w1144) -> ("Output Velocity"=w1141:dbl[])  [unwired: 6 in]
          }
          frame 10 {
            n398 = call "NewVSS_GoTo.vi"("VSSStates"=w1146, "Numeric"=w1145, "Path  Smooth"=w1148, "Position"=w1149, "GoToNavigation?"=w1150) -> ("Output Velocity"=w1147:dbl[])  [unwired: 6 in]
          }
          frame 11 {
            n399 = call "NewVSS_GoTo.vi"("VSSStates"=w1152, "Numeric"=w1151, "Path  Smooth"=w1154, "Position"=w1155, "GoToNavigation?"=w1156) -> ("Output Velocity"=w1153:dbl[])  [unwired: 6 in]
          }
          frame 12 {
            n400 = call "NewVSS_GoTo.vi"("VSSStates"=w1158, "Numeric"=w1157, "Path  Smooth"=w1160, "Position"=w1161, "GoToNavigation?"=w1162) -> ("Output Velocity"=w1159:dbl[])  [unwired: 6 in]
          }
          frame 13 {
            n401 = call "NewVSS_GoTo.vi"("VSSStates"=w1164, "Numeric"=w1163, "Path  Smooth"=w1166, "Position"=w1167, "GoToNavigation?"=w1168) -> ("Output Velocity"=w1165:dbl[])  [unwired: 6 in]
          }
          frame 14 {
            n402 = call "NewVSS_GoTo.vi"("VSSStates"=w1170, "Numeric"=w1169, "Path  Smooth"=w1172, "Position"=w1173, "GoToNavigation?"=w1174) -> ("Output Velocity"=w1171:dbl[])  [unwired: 6 in]
          }
          frame 15 {
            n403 = call "NewVSS_GoTo.vi"("VSSStates"=w1176, "Numeric"=w1175, "Path  Smooth"=w1178, "Position"=w1179, "GoToNavigation?"=w1180) -> ("Output Velocity"=w1177:dbl[])  [unwired: 6 in]
          }
        }
        n404 = Index Array(array=w1077) -> (element #1=w1066:dbl, element #2=w1064:dbl)  [unwired: 2 in]
        n405 = In Range and Coerce(upper limit=0.15, x=w1066, lower limit=w1070) -> (coerced(x)=w1065:dbl)  [unwired: 1 out]
        n406 = In Range and Coerce(upper limit=0.15, x=w1064, lower limit=w1069) -> (coerced(x)=w1063:dbl)  [unwired: 1 out]
        n407 = Bundle By Name(cluster=w1078, "v_tangent"=w1065, "v_normal"=w1063, "v_ang"=0.0) -> (w1075:T3)
      }
      n408 = Bundle By Name(cluster=w1059, "our_robots"=w1058) -> (w1060:T2)
    }
  }
  n409 = Unbundle By Name(w5) -> ("IA Judge.command enum"=w6:T12)
  n410 = Equal?(x=w6, y=Command_Enum."Halt") -> ()  [unwired: 1 out]
  n411 = case shown="True" "Debug" {
    tunnel: [w1181 w1186] -> w4
    tunnel: w5 -> [w1181 w1183]
    tunnel: "IA State Output in" -> [_ w1184]
    frame False {
    }
    frame True {
      n412 = Unbundle By Name(w1183) -> ("our_robots"=w1182:T3[])
      n413 = for {
        tunnel: [w1189] -> w1185 mode=indexing
        tunnel: w1182 -> [w1187] mode=indexing
        w1188 = 0.0 ("v_normal")
        n414 = Bundle By Name(cluster=w1187, "v_tangent"=w1188, "v_normal"=w1188, "v_ang"=w1188) -> (w1189:T3)
      }
      n415 = Bundle By Name(cluster=w1184, "our_robots"=w1185) -> (w1186:T2)
    }
  }
  "IA State Output out" <- w4
